vi "compress_parameters_1.vi"(2 "analog parameters":dbl[](array[numeric]), 3 "AI table":string[](array[string]), 4 "date/time string":string, 5 "table":string) -> (0 "Data to write":bool, 1 "parameters":string)   [LabVIEW 2019, in "PostgreSQL.lvlib"]
uses:
  PostgreSQL.lvlib
panel:
  in  "default string":string="INSERT INTO public.\"XX00.XX00.XX00.XX00.XX00_XQ.7001\"\n (\"time\", \"XX00XX00XX00XX00XX000000_XQ01\", \"XX00XX00XX00XX00XX000001_XQ01\", \"XX00XX00XX00XX00XX000002_XQ01\", \"XX00XX00XX00XX00XX000003_XQ01\", \"XX00XX00XX00XX00XX000004_XQ01\", \"XX00XX00XX00XX00XX000005_XQ01\", \"XX00XX00XX00XX00XX000006_XQ01\", \"XX00XX00XX00XX00XX000007_XQ01\", \"XX00XX00XX00XX00XX000008_XQ01\", \"XX00XX00XX00XX00XX000009_XQ01\", \"XX00XX00XX00XX00XX000010_XQ01\", \"XX00XX00XX00XX00XX000011_XQ01\", \"XX00XX00XX00XX00XX000012_XQ01\", \"XX00XX00XX00XX00XX000013_XQ01\", \"XX00XX00XX00XX00XX000014_XQ01\", \"XX00XX00XX00XX00XX000015_XQ01\", \"XX00XX00XX00XX00XX000016_XQ01\", \"XX00XX00XX00XX00XX000017_XQ01\", \"XX00XX00XX00XX00XX000018_XQ01\", \"XX00XX00XX00XX00XX000019_XQ01\", \"XX00XX00XX00XX00XX000020_XQ01\", \"XX00XX00XX00XX00XX000021_XQ01\", \"XX00XX00XX00XX00XX000022_XQ01\", \"XX00XX00XX00XX00XX000023_XQ01\", \"XX00XX00XX00XX00XX000024_XQ01\", \"XX00XX00XX00XX00XX000025_XQ01\", \"XX00XX00XX00XX00XX000026_XQ01\", \"XX00XX00XX00XX00XX000027_XQ01\", \"XX00XX00XX00XX00XX000028_XQ01\", \"XX00XX00XX00XX00XX000029_XQ01\", \"XX00XX00XX00XX00XX000030_XQ01\", \"XX00XX00XX00XX00XX000031_XQ01\", \"XX00XX00XX00XX00XX000032_XQ01\", \"XX00XX00XX00XX00XX000033_XQ01\", \"XX00XX00XX00XX00XX000034_XQ01\", \"XX00XX00XX00XX00XX000035_XQ01\", \"XX00XX00XX00XX00XX000036_XQ01\", \"XX00XX00XX00XX00XX000037_XQ01\", \"XX00XX00XX00XX00XX000038_XQ01\", \"XX00XX00XX00XX00XX000039_XQ01\", \"XX00XX00XX00XX00XX000040_XQ01\", \"XX00XX00XX00XX00XX000041_XQ01\", \"XX00XX00XX00XX00XX000042_XQ01\", \"XX00XX00XX00XX00XX000043_XQ01\", \"XX00XX00XX00XX00XX000044_XQ01\", \"XX00XX00XX00XX00XX000045_XQ01\", \"XX00XX00XX00XX00XX000046_XQ01\", \"XX00XX00XX00XX00XX000047_XQ01\", \"XX00XX00XX00XX00XX000048_XQ01\", \"XX00XX00XX00XX00XX000049_XQ01\", \"XX00XX00XX00XX00XX000050_XQ01\", \"XX00XX00XX00XX00XX000051_XQ01\", \"XX00XX00XX00XX00XX000052_XQ01\", \"XX00XX00XX00XX00XX000053_XQ01\", \"XX00XX00XX00XX00XX000054_XQ01\", \"XX00XX00XX00XX00XX000055_XQ01\", \"XX00XX00XX00XX00XX000056_XQ01\", \"XX00XX00XX00XX00XX000057_XQ01\", \"XX00XX00XX00XX00XX000058_XQ01\", \"XX00XX00XX00XX00XX000059_XQ01\", \"XX00XX00XX00XX00XX000060_XQ01\", \"XX00XX00XX00XX00XX000061_XQ01\", \"XX00XX00XX00XX00XX000062_XQ01\", \"XX00XX00XX00XX00XX000063_XQ01\", \"XX00XX00XX00XX00XX000064_XQ01\", \"XX00XX00XX00XX00XX000065_XQ01\", \"XX00XX00XX00XX00XX000066_XQ01\", \"XX00XX00XX00XX00XX000067_XQ01\", \"XX00XX00XX00XX00XX000068_XQ01\", \"XX00XX00XX00XX00XX000069_XQ01\", \"XX00XX00XX00XX00XX000070_XQ01\", \"XX00XX00XX00XX00XX000071_XQ01\", \"XX00XX00XX00XX00XX000072_XQ01\", \"XX00XX00XX00XX00XX000073_XQ01\", \"XX00XX00XX00XX00XX000074_XQ01\", \"XX00XX00XX00XX00XX000075_XQ01\", \"XX00XX00XX00XX00XX000076_XQ01\", \"XX00XX00XX00XX00XX000077_XQ01\", \"XX00XX00XX00XX00XX000078_XQ01\", \"XX00XX00XX00XX00XX000079_XQ01\", \"XX00XX00XX00XX00XX000080_XQ01\", \"XX00XX00XX00XX00XX000081_XQ01\", \"XX00XX00XX00XX00XX000082_XQ01\", \"XX00XX00XX00XX00XX000083_XQ01\", \"XX00XX00XX00XX00XX000084_XQ01\", \"XX00XX00XX00XX00XX000085_XQ01\", \"XX00XX00XX00XX00XX000086_XQ01\", \"XX00XX00XX00XX00XX000087_XQ01\", \"XX00XX00XX00XX00XX000088_XQ01\", \"XX00XX00XX00XX00XX000089_XQ01\", \"XX00XX00XX00XX00XX000090_XQ01\", \"XX00XX00XX00XX00XX000091_XQ01\", \"XX00XX00XX00XX00XX000092_XQ01\", \"XX00XX00XX00XX00XX000093_XQ01\", \"XX00XX00XX00XX00XX000094_XQ01\", \"XX00XX00XX00XX00XX000095_XQ01\", \"XX00XX00XX00XX00XX000096_XQ01\", \"XX00XX00XX00XX00XX000097_XQ01\", \"XX00XX00XX00XX00XX000098_XQ01\", \"XX00XX00XX00XX00XX000099_XQ01\", \"XX00XX00XX00XX00XX000100_XQ01\", \"XX00XX00XX00XX00XX000101_XQ01\", \"XX00XX00XX00XX00XX000102_XQ01\", \"XX00XX00XX00XX00XX000103_XQ01\", \"XX00XX00XX00XX00XX000104_XQ01\", \"XX00XX00XX00XX00XX000105_XQ01\", \"XX00XX00XX00XX00XX000106_XQ01\", \"XX00XX00XX00XX00XX000107_XQ01\", \"XX00XX00XX00XX00XX000108_XQ01\", \"XX00XX00XX00XX00XX000109_XQ01\", \"XX00XX00XX00XX00XX000110_XQ01\", \"XX00XX00XX00XX00XX000111_XQ01\", \"XX00XX00XX00XX00XX000112_XQ01\", \"XX00XX00XX00XX00XX000113_XQ01\", \"XX00XX00XX00XX00XX000114_XQ01\", \"XX00XX00XX00XX00XX000115_XQ01\", \"XX00XX00XX00XX00XX000116_XQ01\", \"XX00XX00XX00XX00XX000117_XQ01\", \"XX00XX00XX00XX00XX000118_XQ01\", \"XX00XX00XX00XX00XX000119_XQ01\", \"XX00XX00XX00XX00XX000120_XQ01\", \"XX00XX00XX00XX00XX000121_XQ01\", \"XX00XX00XX00XX00XX000122_XQ01\", \"XX00XX00XX00XX00XX000123_XQ01\", \"XX00XX00XX00XX00XX000124_XQ01\", \"XX00XX00XX00XX00XX000125_XQ01\", \"XX00XX00XX00XX00XX000126_XQ01\", \"XX00XX00XX00XX00XX000127_XQ01\", \"XX00XX00XX00XX00XX000128_XQ01\", \"XX00XX00XX00XX00XX000129_XQ01\", \"XX00XX00XX00XX00XX000130_XQ01\", \"XX00XX00XX00XX00XX000131_XQ01\", \"XX00XX00XX00XX00XX000132_XQ01\", \"XX00XX00XX00XX00XX000133_XQ01\", \"XX00XX00XX00XX00XX000134_XQ01\", \"XX00XX00XX00XX00XX000135_XQ01\", \"XX00XX00XX00XX00XX000136_XQ01\", \"XX00XX00XX00XX00XX000137_XQ01\", \"XX00XX00XX00XX00XX000138_XQ01\", \"XX00XX00XX00XX00XX000139_XQ01\", \"XX00XX00XX00XX00XX000140_XQ01\", \"XX00XX00XX00XX00XX000141_XQ01\", \"XX00XX00XX00XX00XX000142_XQ01\", \"XX00XX00XX00XX00XX000143_XQ01\", \"XX00XX00XX00XX00XX000144_XQ01\", \"XX00XX00XX00XX00XX000145_XQ01\", \"XX00XX00XX00XX00XX000146_XQ01\", \"XX00XX00XX00XX00XX000147_XQ01\", \"XX00XX00XX00XX00XX000148_XQ01\", \"XX00XX00XX00XX00XX000149_XQ01\", \"XX00XX00XX00XX00XX000150_XQ01\", \"XX00XX00XX00XX00XX000151_XQ01\", \"XX00XX00XX00XX00XX000152_XQ01\", \"XX00XX00XX00XX00XX000153_XQ01\", \"XX00XX00XX00XX00XX000154_XQ01\", \"XX00XX00XX00XX00XX000155_XQ01\", \"XX00XX00XX00XX00XX000156_XQ01\", \"XX00XX00XX00XX00XX000157_XQ01\", \"XX00XX00XX00XX00XX000158_XQ01\", \"XX00XX00XX00XX00XX000159_XQ01\", \"XX00XX00XX00XX00XX000160_XQ01\", \"XX00XX00XX00XX00XX000161_XQ01\", \"XX00XX00XX00XX00XX000162_XQ01\", \"XX00XX00XX00XX00XX000163_XQ01\", \"XX00XX00XX00XX00XX000164_XQ01\", \"XX00XX00XX00XX00XX000165_XQ01\", \"XX00XX00XX00XX00XX000166_XQ01\", \"XX00XX00XX00XX00XX000167_XQ01\", \"XX00XX00XX00XX00XX000168_XQ01\", \"XX00XX00XX00XX00XX000169_XQ01\", \"XX00XX00XX00XX00XX000170_XQ01\", \"XX00XX00XX00XX00XX000171_XQ01\", \"XX00XX00XX00XX00XX000172_XQ01\", \"XX00XX00XX00XX00XX000173_XQ01\", \"XX00XX00XX00XX00XX000174_XQ01\", \"XX00XX00XX00XX00XX000175_XQ01\", \"XX00XX00XX00XX00XX000176_XQ01\", \"XX00XX00XX00XX00XX000177_XQ01\", \"XX00XX00XX00XX00XX000178_XQ01\", \"XX00XX00XX00XX00XX000179_XQ01\", \"XX00XX00XX00XX00XX000180_XQ01\", \"XX00XX00XX00XX00XX000181_XQ01\", \"XX00XX00XX00XX00XX000182_XQ01\", \"XX00XX00XX00XX00XX000183_XQ01\", \"XX00XX00XX00XX00XX000184_XQ01\", \"XX00XX00XX00XX00XX000185_XQ01\", \"XX00XX00XX00XX00XX000186_XQ01\", \"XX00XX00XX00XX00XX000187_XQ01\", \"XX00XX00XX00XX00XX000188_XQ01\", \"XX00XX00XX00XX00XX000189_XQ01\", \"XX00XX00XX00XX00XX000190_XQ01\", \"XX00XX00XX00XX00XX000191_XQ01\", \"XX00XX00XX00XX00XX000192_XQ01\", \"XX00XX00XX00XX00XX000193_XQ01\", \"XX00XX00XX00XX00XX000194_XQ01\", \"XX00XX00XX00XX00XX000195_XQ01\", \"XX00XX00XX00XX00XX000196_XQ01\", \"XX00XX00XX00XX00XX000197_XQ01\", \"XX00XX00XX00XX00XX000198_XQ01\", \"XX00XX00XX00XX00XX000199_XQ01\", \"XX00XX00XX00XX00XX000200_XQ01\", \"XX00XX00XX00XX00XX000201_XQ01\", \"XX00XX00XX00XX00XX000202_XQ01\", \"XX00XX00XX00XX00XX000203_XQ01\", \"XX00XX00XX00XX00XX000204_XQ01\", \"XX00XX00XX00XX00XX000205_XQ01\", \"XX00XX00XX00XX00XX000206_XQ01\", \"XX00XX00XX00XX00XX000207_XQ01\", \"XX00XX00XX00XX00XX000208_XQ01\", \"XX00XX00XX00XX00XX000209_XQ01\", \"XX00XX00XX00XX00XX000210_XQ01\", \"XX00XX00XX00XX00XX000211_XQ01\", \"XX00XX00XX00XX00XX000212_XQ01\", \"XX00XX00XX00XX00XX000213_XQ01\", \"XX00XX00XX00XX00XX000214_XQ01\", \"XX00XX00XX00XX00XX000215_XQ01\", \"XX00XX00XX00XX00XX000216_XQ01\", \"XX00XX00XX00XX00XX000217_XQ01\", \"XX00XX00XX00XX00XX000218_XQ01\", \"XX00XX00XX00XX00XX000219_XQ01\", \"XX00XX00XX00XX00XX000220_XQ01\", \"XX00XX00XX00XX00XX000221_XQ01\", \"XX00XX00XX00XX00XX000222_XQ01\", \"XX00XX00XX00XX00XX000223_XQ01\", \"XX00XX00XX00XX00XX000224_XQ01\", \"XX00XX00XX00XX00XX000225_XQ01\", \"XX00XX00XX00XX00XX000226_XQ01\", \"XX00XX00XX00XX00XX000227_XQ01\", \"XX00XX00XX00XX00XX000228_XQ01\", \"XX00XX00XX00XX00XX000229_XQ01\", \"XX00XX00XX00XX00XX000230_XQ01\", \"XX00XX00XX00XX00XX000231_XQ01\", \"XX00XX00XX00XX00XX000232_XQ01\", \"XX00XX00XX00XX00XX000233_XQ01\", \"XX00XX00XX00XX00XX000234_XQ01\", \"XX00XX00XX00XX00XX000235_XQ01\", \"XX00XX00XX00XX00XX000236_XQ01\", \"XX00XX00XX00XX00XX000237_XQ01\", \"XX00XX00XX00XX00XX000238_XQ01\", \"XX00XX00XX00XX00XX000239_XQ01\", \"XX00XX00XX00XX00XX000240_XQ01\", \"XX00XX00XX00XX00XX000241_XQ01\", \"XX00XX00XX00XX00XX000242_XQ01\", \"XX00XX00XX00XX00XX000243_XQ01\", \"XX00XX00XX00XX00XX000244_XQ01\", \"XX00XX00XX00XX00XX000245_XQ01\", \"XX00XX00XX00XX00XX000246_XQ01\", \"XX00XX00XX00XX00XX000247_XQ01\", \"XX00XX00XX00XX00XX000248_XQ01\", \"XX00XX00XX00XX00XX000249_XQ01\", \"XX00XX00XX00XX00XX000250_XQ01\", \"XX00XX00XX00XX00XX000251_XQ01\", \"XX00XX00XX00XX00XX000252_XQ01\", \"XX00XX00XX00XX00XX000253_XQ01\", \"XX00XX00XX00XX00XX000254_XQ01\", \"XX00XX00XX00XX00XX000255_XQ01\", \"XX00XX00XX00XX00XX000256_XQ01\", \"XX00XX00XX00XX00XX000257_XQ01\", \"XX00XX00XX00XX00XX000258_XQ01\", \"XX00XX00XX00XX00XX000259_XQ01\", \"XX00XX00XX00XX00XX000260_XQ01\", \"XX00XX00XX00XX00XX000261_XQ01\", \"XX00XX00XX00XX00XX000262_XQ01\", \"XX00XX00XX00XX00XX000263_XQ01\", \"XX00XX00XX00XX00XX000264_XQ01\", \"XX00XX00XX00XX00XX000265_XQ01\", \"XX00XX00XX00XX00XX000266_XQ01\", \"XX00XX00XX00XX00XX000267_XQ01\", \"XX00XX00XX00XX00XX000268_XQ01\", \"XX00XX00XX00XX00XX000269_XQ01\", \"XX00XX00XX00XX00XX000270_XQ01\", \"XX00XX00XX00XX00XX000271_XQ01\", \"XX00XX00XX00XX00XX000272_XQ01\", \"XX00XX00XX00XX00XX000273_XQ01\", \"XX00XX00XX00XX00XX000274_XQ01\", \"XX00XX00XX00XX00XX000275_XQ01\", \"XX00XX00XX00XX00XX000276_XQ01\", \"XX00XX00XX00XX00XX000277_XQ01\", \"XX00XX00XX00XX00XX000278_XQ01\", \"XX00XX00XX00XX00XX000279_XQ01\", \"XX00XX00XX00XX00XX000280_XQ01\", \"XX00XX00XX00XX00XX000281_XQ01\", \"XX00XX00XX00XX00XX000282_XQ01\", \"XX00XX00XX00XX00XX000283_XQ01\", \"XX00XX00XX00XX00XX000284_XQ01\", \"XX00XX00XX00XX00XX000285_XQ01\", \"XX00XX00XX00XX00XX000286_XQ01\", \"XX00XX00XX00XX00XX000287_XQ01\", \"XX00XX00XX00XX00XX000288_XQ01\", \"XX00XX00XX00XX00XX000289_XQ01\", \"XX00XX00XX00XX00XX000290_XQ01\", \"XX00XX00XX00XX00XX000291_XQ01\", \"XX00XX00XX00XX00XX000292_XQ01\", \"XX00XX00XX00XX00XX000293_XQ01\", \"XX00XX00XX00XX00XX000294_XQ01\", \"XX00XX00XX00XX00XX000295_XQ01\", \"XX00XX00XX00XX00XX000296_XQ01\", \"XX00XX00XX00XX00XX000297_XQ01\", \"XX00XX00XX00XX00XX000298_XQ01\", \"XX00XX00XX00XX00XX000299_XQ01\", \"XX00XX00XX00XX00XX000300_XQ01\", \"XX00XX00XX00XX00XX000301_XQ01\", \"XX00XX00XX00XX00XX000302_XQ01\", \"XX00XX00XX00XX00XX000303_XQ01\", \"XX00XX00XX00XX00XX000304_XQ01\", \"XX00XX00XX00XX00XX000305_XQ01\", \"XX00XX00XX00XX00XX000306_XQ01\", \"XX00XX00XX00XX00XX000307_XQ01\", \"XX00XX00XX00XX00XX000308_XQ01\", \"XX00XX00XX00XX00XX000309_XQ01\", \"XX00XX00XX00XX00XX000310_XQ01\", \"XX00XX00XX00XX00XX000311_XQ01\", \"XX00XX00XX00XX00XX000312_XQ01\", \"XX00XX00XX00XX00XX000313_XQ01\", \"XX00XX00XX00XX00XX000314_XQ01\", \"XX00XX00XX00XX00XX000315_XQ01\", \"XX00XX00XX00XX00XX000316_XQ01\", \"XX00XX00XX00XX00XX000317_XQ01\", \"XX00XX00XX00XX00XX000318_XQ01\", \"XX00XX00XX00XX00XX000319_XQ01\", \"XX00XX00XX00XX00XX000320_XQ01\", \"XX00XX00XX00XX00XX000321_XQ01\", \"XX00XX00XX00XX00XX000322_XQ01\", \"XX00XX00XX00XX00XX000323_XQ01\", \"XX00XX00XX00XX00XX000324_XQ01\", \"XX00XX00XX00XX00XX000325_XQ01\", \"XX00XX00XX00XX00XX000326_XQ01\", \"XX00XX00XX00XX00XX000327_XQ01\", \"XX00XX00XX00XX00XX000328_XQ01\", \"XX00XX00XX00XX00XX000329_XQ01\", \"XX00XX00XX00XX00XX000330_XQ01\", \"XX00XX00XX00XX00XX000331_XQ01\", \"XX00XX00XX00XX00XX000332_XQ01\", \"XX00XX00XX00XX00XX000333_XQ01\", \"XX00XX00XX00XX00XX000334_XQ01\", \"XX00XX00XX00XX00XX000335_XQ01\", \"XX00XX00XX00XX00XX000336_XQ01\", \"XX00XX00XX00XX00XX000337_XQ01\", \"XX00XX00XX00XX00XX000338_XQ01\", \"XX00XX00XX00XX00XX000339_XQ01\", \"XX00XX00XX00XX00XX000340_XQ01\", \"XX00XX00XX00XX00XX000341_XQ01\", \"XX00XX00XX00XX00XX000342_XQ01\", \"XX00XX00XX00XX00XX000343_XQ01\", \"XX00XX00XX00XX00XX000344_XQ01\", \"XX00XX00XX00XX00XX000345_XQ01\", \"XX00XX00XX00XX00XX000346_XQ01\", \"XX00XX00XX00XX00XX000347_XQ01\", \"XX00XX00XX00XX00XX000348_XQ01\", \"XX00XX00XX00XX00XX000349_XQ01\", \"XX00XX00XX00XX00XX000350_XQ01\", \"XX00XX00XX00XX00XX000351_XQ01\", \"XX00XX00XX00XX00XX000352_XQ01\", \"XX00XX00XX00XX00XX000353_XQ01\", \"XX00XX00XX00XX00XX000354_XQ01\", \"XX00XX00XX00XX00XX000355_XQ01\", \"XX00XX00XX00XX00XX000356_XQ01\", \"XX00XX00XX00XX00XX000357_XQ01\", \"XX00XX00XX00XX00XX000358_XQ01\", \"XX00XX00XX00XX00XX000359_XQ01\", \"XX00XX00XX00XX00XX000360_XQ01\", \"XX00XX00XX00XX00XX000361_XQ01\", \"XX00XX00XX00XX00XX000362_XQ01\", \"XX00XX00XX00XX00XX000363_XQ01\", \"XX00XX00XX00XX00XX000364_XQ01\", \"XX00XX00XX00XX00XX000365_XQ01\", \"XX00XX00XX00XX00XX000366_XQ01\", \"XX00XX00XX00XX00XX000367_XQ01\", \"XX00XX00XX00XX00XX000368_XQ01\", \"XX00XX00XX00XX00XX000369_XQ01\", \"XX00XX00XX00XX00XX000370_XQ01\", \"XX00XX00XX00XX00XX000371_XQ01\", \"XX00XX00XX00XX00XX000372_XQ01\", \"XX00XX00XX00XX00XX000373_XQ01\", \"XX00XX00XX00XX00XX000374_XQ01\", \"XX00XX00XX00XX00XX000375_XQ01\", \"XX00XX00XX00XX00XX000376_XQ01\", \"XX00XX00XX00XX00XX000377_XQ01\", \"XX00XX00XX00XX00XX000378_XQ01\", \"XX00XX00XX00XX00XX000379_XQ01\", \"XX00XX00XX00XX00XX000380_XQ01\", \"XX00XX00XX00XX00XX000381_XQ01\", \"XX00XX00XX00XX00XX000382_XQ01\", \"XX00XX00XX00XX00XX000383_XQ01\", \"XX00XX00XX00XX00XX000384_XQ01\", \"XX00XX00XX00XX00XX000385_XQ01\", \"XX00XX00XX00XX00XX000386_XQ01\", \"XX00XX00XX00XX00XX000387_XQ01\", \"XX00XX00XX00XX00XX000388_XQ01\", \"XX00XX00XX00XX00XX000389_XQ01\", \"XX00XX00XX00XX00XX000390_XQ01\", \"XX00XX00XX00XX00XX000391_XQ01\", \"XX00XX00XX00XX00XX000392_XQ01\", \"XX00XX00XX00XX00XX000393_XQ01\", \"XX00XX00XX00XX00XX000394_XQ01\", \"XX00XX00XX00XX00XX000395_XQ01\", \"XX00XX00XX00XX00XX000396_XQ01\", \"XX00XX00XX00XX00XX000397_XQ01\", \"XX00XX00XX00XX00XX000398_XQ01\", \"XX00XX00XX00XX00XX000399_XQ01\", \"XX00XX00XX00XX00XX000400_XQ01\", \"XX00XX00XX00XX00XX000401_XQ01\", \"XX00XX00XX00XX00XX000402_XQ01\", \"XX00XX00XX00XX00XX000403_XQ01\", \"XX00XX00XX00XX00XX000404_XQ01\", \"XX00XX00XX00XX00XX000405_XQ01\", \"XX00XX00XX00XX00XX000406_XQ01\", \"XX00XX00XX00XX00XX000407_XQ01\", \"XX00XX00XX00XX00XX000408_XQ01\", \"XX00XX00XX00XX00XX000409_XQ01\", \"XX00XX00XX00XX00XX000410_XQ01\", \"XX00XX00XX00XX00XX000411_XQ01\", \"XX00XX00XX00XX00XX000412_XQ01\", \"XX00XX00XX00XX00XX000413_XQ01\", \"XX00XX00XX00XX00XX000414_XQ01\", \"XX00XX00XX00XX00XX000415_XQ01\", \"XX00XX00XX00XX00XX000416_XQ01\", \"XX00XX00XX00XX00XX000417_XQ01\", \"XX00XX00XX00XX00XX000418_XQ01\", \"XX00XX00XX00XX00XX000419_XQ01\", \"XX00XX00XX00XX00XX000420_XQ01\", \"XX00XX00XX00XX00XX000421_XQ01\", \"XX00XX00XX00XX00XX000422_XQ01\", \"XX00XX00XX00XX00XX000423_XQ01\", \"XX00XX00XX00XX00XX000424_XQ01\", \"XX00XX00XX00XX00XX000425_XQ01\", \"XX00XX00XX00XX00XX000426_XQ01\", \"XX00XX00XX00XX00XX000427_XQ01\", \"XX00XX00XX00XX00XX000428_XQ01\", \"XX00XX00XX00XX00XX000429_XQ01\", \"XX00XX00XX00XX00XX000430_XQ01\", \"XX00XX00XX00XX00XX000431_XQ01\", \"XX00XX00XX00XX00XX000432_XQ01\", \"XX00XX00XX00XX00XX000433_XQ01\", \"XX00XX00XX00XX00XX000434_XQ01\", \"XX00XX00XX00XX00XX000435_XQ01\", \"XX00XX00XX00XX00XX000436_XQ01\", \"XX00XX00XX00XX00XX000437_XQ01\", \"XX00XX00XX00XX00XX000438_XQ01\", \"XX00XX00XX00XX00XX000439_XQ01\", \"XX00XX00XX00XX00XX000440_XQ01\", \"XX00XX00XX00XX00XX000441_XQ01\", \"XX00XX00XX00XX00XX000442_XQ01\", \"XX00XX00XX00XX00XX000443_XQ01\", \"XX00XX00XX00XX00XX000444_XQ01\", \"XX00XX00XX00XX00XX000445_XQ01\", \"XX00XX00XX00XX00XX000446_XQ01\", \"XX00XX00XX00XX00XX000447_XQ01\", \"XX00XX00XX00XX00XX000448_XQ01\", \"XX00XX00XX00XX00XX000449_XQ01\", \"XX00XX00XX00XX00XX000450_XQ01\", \"XX00XX00XX00XX00XX000451_XQ01\", \"XX00XX00XX00XX00XX000452_XQ01\", \"XX00XX00XX00XX00XX000453_XQ01\", \"XX00XX00XX00XX00XX000454_XQ01\", \"XX00XX00XX00XX00XX000455_XQ01\", \"XX00XX00XX00XX00XX000456_XQ01\", \"XX00XX00XX00XX00XX000457_XQ01\", \"XX00XX00XX00XX00XX000458_XQ01\", \"XX00XX00XX00XX00XX000459_XQ01\", \"XX00XX00XX00XX00XX000460_XQ01\", \"XX00XX00XX00XX00XX000461_XQ01\", \"XX00XX00XX00XX00XX000462_XQ01\", \"XX00XX00XX00XX00XX000463_XQ01\", \"XX00XX00XX00XX00XX000464_XQ01\", \"XX00XX00XX00XX00XX000465_XQ01\", \"XX00XX00XX00XX00XX000466_XQ01\", \"XX00XX00XX00XX00XX000467_XQ01\", \"XX00XX00XX00XX00XX000468_XQ01\", \"XX00XX00XX00XX00XX000469_XQ01\", \"XX00XX00XX00XX00XX000470_XQ01\", \"XX00XX00XX00XX00XX000471_XQ01\", \"XX00XX00XX00XX00XX000472_XQ01\", \"XX00XX00XX00XX00XX000473_XQ01\", \"XX00XX00XX00XX00XX000474_XQ01\", \"XX00XX00XX00XX00XX000475_XQ01\", \"XX00XX00XX00XX00XX000476_XQ01\", \"XX00XX00XX00XX00XX000477_XQ01\", \"XX00XX00XX00XX00XX000478_XQ01\", \"XX00XX00XX00XX00XX000479_XQ01\", \"XX00XX00XX00XX00XX000480_XQ01\", \"XX00XX00XX00XX00XX000481_XQ01\", \"XX00XX00XX00XX00XX000482_XQ01\", \"XX00XX00XX00XX00XX000483_XQ01\", \"XX00XX00XX00XX00XX000484_XQ01\", \"XX00XX00XX00XX00XX000485_XQ01\", \"XX00XX00XX00XX00XX000486_XQ01\", \"XX00XX00XX00XX00XX000487_XQ01\", \"XX00XX00XX00XX00XX000488_XQ01\", \"XX00XX00XX00XX00XX000489_XQ01\", \"XX00XX00XX00XX00XX000490_XQ01\", \"XX00XX00XX00XX00XX000491_XQ01\", \"XX00XX00XX00XX00XX000492_XQ01\", \"XX00XX00XX00XX00XX000493_XQ01\", \"XX00XX00XX00XX00XX000494_XQ01\", \"XX00XX00XX00XX00XX000495_XQ01\", \"XX00XX00XX00XX00XX000496_XQ01\", \"XX00XX00XX00XX00XX000497_XQ01\", \"XX00XX00XX00XX00XX000498_XQ01\", \"XX00XX00XX00XX00XX000499_XQ01\", \"XX00XX00XX00XX00XX000500_XQ01\", \"XX00XX00XX00XX00XX000501_XQ01\", \"XX00XX00XX00XX00XX000502_XQ01\", \"XX00XX00XX00XX00XX000503_XQ01\", \"XX00XX00XX00XX00XX000504_XQ01\", \"XX00XX00XX00XX00XX000505_XQ01\", \"XX00XX00XX00XX00XX000506_XQ01\", \"XX00XX00XX00XX00XX000507_XQ01\", \"XX00XX00XX00XX00XX000508_XQ01\", \"XX00XX00XX00XX00XX000509_XQ01\", \"XX00XX00XX00XX00XX000510_XQ01\", \"XX00XX00XX00XX00XX000511_XQ01\", \"XX00XX00XX00XX00XX000512_XQ01\", \"XX00XX00XX00XX00XX000513_XQ01\", \"XX00XX00XX00XX00XX000514_XQ01\", \"XX00XX00XX00XX00XX000515_XQ01\", \"XX00XX00XX00XX00XX000516_XQ01\", \"XX00XX00XX00XX00XX000517_XQ01\", \"XX00XX00XX00XX00XX000518_XQ01\", \"XX00XX00XX00XX00XX000519_XQ01\", \"XX00XX00XX00XX00XX000520_XQ01\", \"XX00XX00XX00XX00XX000521_XQ01\", \"XX00XX00XX00XX00XX000522_XQ01\", \"XX00XX00XX00XX00XX000523_XQ01\", \"XX00XX00XX00XX00XX000524_XQ01\", \"XX00XX00XX00XX00XX000525_XQ01\", \"XX00XX00XX00XX00XX000526_XQ01\", \"XX00XX00XX00XX00XX000527_XQ01\", \"XX00XX00XX00XX00XX000528_XQ01\", \"XX00XX00XX00XX00XX000529_XQ01\", \"XX00XX00XX00XX00XX000530_XQ01\", \"XX00XX00XX00XX00XX000531_XQ01\", \"XX00XX00XX00XX00XX000532_XQ01\", \"XX00XX00XX00XX00XX000533_XQ01\", \"XX00XX00XX00XX00XX000534_XQ01\", \"XX00XX00XX00XX00XX000535_XQ01\", \"XX00XX00XX00XX00XX000536_XQ01\", \"XX00XX00XX00XX00XX000537_XQ01\", \"XX00XX00XX00XX00XX000538_XQ01\", \"XX00XX00XX00XX00XX000539_XQ01\", \"XX00XX00XX00XX00XX000540_XQ01\", \"XX00XX00XX00XX00XX000541_XQ01\", \"XX00XX00XX00XX00XX000542_XQ01\", \"XX00XX00XX00XX00XX000543_XQ01\", \"XX00XX00XX00XX00XX000544_XQ01\", \"XX00XX00XX00XX00XX000545_XQ01\", \"XX00XX00XX00XX00XX000546_XQ01\", \"XX00XX00XX00XX00XX000547_XQ01\", \"XX00XX00XX00XX00XX000548_XQ01\", \"XX00XX00XX00XX00XX000549_XQ01\", \"XX00XX00XX00XX00XX000550_XQ01\", \"XX00XX00XX00XX00XX000551_XQ01\", \"XX00XX00XX00XX00XX000552_XQ01\", \"XX00XX00XX00XX00XX000553_XQ01\", \"XX00XX00XX00XX00XX000554_XQ01\", \"XX00XX00XX00XX00XX000555_XQ01\", \"XX00XX00XX00XX00XX000556_XQ01\", \"XX00XX00XX00XX00XX000557_XQ01\", \"XX00XX00XX00XX00XX000558_XQ01\", \"XX00XX00XX00XX00XX000559_XQ01\", \"XX00XX00XX00XX00XX000560_XQ01\", \"XX00XX00XX00XX00XX000561_XQ01\", \"XX00XX00XX00XX00XX000562_XQ01\", \"XX00XX00XX00XX00XX000563_XQ01\", \"XX00XX00XX00XX00XX000564_XQ01\", \"XX00XX00XX00XX00XX000565_XQ01\", \"XX00XX00XX00XX00XX000566_XQ01\", \"XX00XX00XX00XX00XX000567_XQ01\", \"XX00XX00XX00XX00XX000568_XQ01\", \"XX00XX00XX00XX00XX000569_XQ01\", \"XX00XX00XX00XX00XX000570_XQ01\", \"XX00XX00XX00XX00XX000571_XQ01\", \"XX00XX00XX00XX00XX000572_XQ01\", \"XX00XX00XX00XX00XX000573_XQ01\", \"XX00XX00XX00XX00XX000574_XQ01\", \"XX00XX00XX00XX00XX000575_XQ01\", \"XX00XX00XX00XX00XX000576_XQ01\", \"XX00XX00XX00XX00XX000577_XQ01\", \"XX00XX00XX00XX00XX000578_XQ01\", \"XX00XX00XX00XX00XX000579_XQ01\", \"XX00XX00XX00XX00XX000580_XQ01\", \"XX00XX00XX00XX00XX000581_XQ01\", \"XX00XX00XX00XX00XX000582_XQ01\", \"XX00XX00XX00XX00XX000583_XQ01\", \"XX00XX00XX00XX00XX000584_XQ01\", \"XX00XX00XX00XX00XX000585_XQ01\", \"XX00XX00XX00XX00XX000586_XQ01\", \"XX00XX00XX00XX00XX000587_XQ01\", \"XX00XX00XX00XX00XX000588_XQ01\", \"XX00XX00XX00XX00XX000589_XQ01\", \"XX00XX00XX00XX00XX000590_XQ01\", \"XX00XX00XX00XX00XX000591_XQ01\", \"XX00XX00XX00XX00XX000592_XQ01\", \"XX00XX00XX00XX00XX000593_XQ01\", \"XX00XX00XX00XX00XX000594_XQ01\", \"XX00XX00XX00XX00XX000595_XQ01\", \"XX00XX00XX00XX00XX000596_XQ01\", \"XX00XX00XX00XX00XX000597_XQ01\", \"XX00XX00XX00XX00XX000598_XQ01\", \"XX00XX00XX00XX00XX000599_XQ01\", \"XX00XX00XX00XX00XX000600_XQ01\", \"XX00XX00XX00XX00XX000601_XQ01\", \"XX00XX00XX00XX00XX000602_XQ01\", \"XX00XX00XX00XX00XX000603_XQ01\", \"XX00XX00XX00XX00XX000604_XQ01\", \"XX00XX00XX00XX00XX000605_XQ01\", \"XX00XX00XX00XX00XX000606_XQ01\", \"XX00XX00XX00XX00XX000607_XQ01\", \"XX00XX00XX00XX00XX000608_XQ01\", \"XX00XX00XX00XX00XX000609_XQ01\", \"XX00XX00XX00XX00XX000610_XQ01\", \"XX00XX00XX00XX00XX000611_XQ01\", \"XX00XX00XX00XX00XX000612_XQ01\", \"XX00XX00XX00XX00XX000613_XQ01\", \"XX00XX00XX00XX00XX000614_XQ01\", \"XX00XX00XX00XX00XX000615_XQ01\", \"XX00XX00XX00XX00XX000616_XQ01\", \"XX00XX00XX00XX00XX000617_XQ01\", \"XX00XX00XX00XX00XX000618_XQ01\", \"XX00XX00XX00XX00XX000619_XQ01\", \"XX00XX00XX00XX00XX000620_XQ01\", \"XX00XX00XX00XX00XX000621_XQ01\", \"XX00XX00XX00XX00XX000622_XQ01\", \"XX00XX00XX00XX00XX000623_XQ01\", \"XX00XX00XX00XX00XX000624_XQ01\", \"XX00XX00XX00XX00XX000625_XQ01\", \"XX00XX00XX00XX00XX000626_XQ01\", \"XX00XX00XX00XX00XX000627_XQ01\", \"XX00XX00XX00XX00XX000628_XQ01\", \"XX00XX00XX00XX00XX000629_XQ01\", \"XX00XX00XX00XX00XX000630_XQ01\", \"XX00XX00XX00XX00XX000631_XQ01\", \"XX00XX00XX00XX00XX000632_XQ01\", \"XX00XX00XX00XX00XX000633_XQ01\", \"XX00XX00XX00XX00XX000634_XQ01\", \"XX00XX00XX00XX00XX000635_XQ01\", \"XX00XX00XX00XX00XX000636_XQ01\", \"XX00XX00XX00XX00XX000637_XQ01\", \"XX00XX00XX00XX00XX000638_XQ01\", \"XX00XX00XX00XX00XX000639_XQ01\", \"XX00XX00XX00XX00XX000640_XQ01\", \"XX00XX00XX00XX00XX000641_XQ01\", \"XX00XX00XX00XX00XX000642_XQ01\", \"XX00XX00XX00XX00XX000643_XQ01\", \"XX00XX00XX00XX00XX000644_XQ01\", \"XX00XX00XX00XX00XX000645_XQ01\", \"XX00XX00XX00XX00XX000646_XQ01\", \"XX00XX00XX00XX00XX000647_XQ01\", \"XX00XX00XX00XX00XX000648_XQ01\", \"XX00XX00XX00XX00XX000649_XQ01\", \"XX00XX00XX00XX00XX000650_XQ01\", \"XX00XX00XX00XX00XX000651_XQ01\", \"XX00XX00XX00XX00XX000652_XQ01\", \"XX00XX00XX00XX00XX000653_XQ01\", \"XX00XX00XX00XX00XX000654_XQ01\", \"XX00XX00XX00XX00XX000655_XQ01\", \"XX00XX00XX00XX00XX000656_XQ01\", \"XX00XX00XX00XX00XX000657_XQ01\", \"XX00XX00XX00XX00XX000658_XQ01\", \"XX00XX00XX00XX00XX000659_XQ01\", \"XX00XX00XX00XX00XX000660_XQ01\", \"XX00XX00XX00XX00XX000661_XQ01\", \"XX00XX00XX00XX00XX000662_XQ01\", \"XX00XX00XX00XX00XX000663_XQ01\", \"XX00XX00XX00XX00XX000664_XQ01\", \"XX00XX00XX00XX00XX000665_XQ01\", \"XX00XX00XX00XX00XX000666_XQ01\", \"XX00XX00XX00XX00XX000667_XQ01\", \"XX00XX00XX00XX00XX000668_XQ01\", \"XX00XX00XX00XX00XX000669_XQ01\", \"XX00XX00XX00XX00XX000670_XQ01\", \"XX00XX00XX00XX00XX000671_XQ01\", \"XX00XX00XX00XX00XX000672_XQ01\", \"XX00XX00XX00XX00XX000673_XQ01\", \"XX00XX00XX00XX00XX000674_XQ01\", \"XX00XX00XX00XX00XX000675_XQ01\", \"XX00XX00XX00XX00XX000676_XQ01\", \"XX00XX00XX00XX00XX000677_XQ01\", \"XX00XX00XX00XX00XX000678_XQ01\", \"XX00XX00XX00XX00XX000679_XQ01\", \"XX00XX00XX00XX00XX000680_XQ01\", \"XX00XX00XX00XX00XX000681_XQ01\", \"XX00XX00XX00XX00XX000682_XQ01\", \"XX00XX00XX00XX00XX000683_XQ01\", \"XX00XX00XX00XX00XX000684_XQ01\", \"XX00XX00XX00XX00XX000685_XQ01\", \"XX00XX00XX00XX00XX000686_XQ01\", \"XX00XX00XX00XX00XX000687_XQ01\", \"XX00XX00XX00XX00XX000688_XQ01\", \"XX00XX00XX00XX00XX000689_XQ01\", \"XX00XX00XX00XX00XX000690_XQ01\", \"XX00XX00XX00XX00XX000691_XQ01\", \"XX00XX00XX00XX00XX000692_XQ01\", \"XX00XX00XX00XX00XX000693_XQ01\", \"XX00XX00XX00XX00XX000694_XQ01\", \"XX00XX00XX00XX00XX000695_XQ01\", \"XX00XX00XX00XX00XX000696_XQ01\", \"XX00XX00XX00XX00XX000697_XQ01\", \"XX00XX00XX00XX00XX000698_XQ01\", \"XX00XX00XX00XX00XX000699_XQ01\", \"XX00XX00XX00XX00XX000700_XQ01\", \"XX00XX00XX00XX00XX000701_XQ01\", \"XX00XX00XX00XX00XX000702_XQ01\", \"XX00XX00XX00XX00XX000703_XQ01\", \"XX00XX00XX00XX00XX000704_XQ01\", \"XX00XX00XX00XX00XX000705_XQ01\", \"XX00XX00XX00XX00XX000706_XQ01\", \"XX00XX00XX00XX00XX000707_XQ01\", \"XX00XX00XX00XX00XX000708_XQ01\", \"XX00XX00XX00XX00XX000709_XQ01\", \"XX00XX00XX00XX00XX000710_XQ01\", \"XX00XX00XX00XX00XX000711_XQ01\", \"XX00XX00XX00XX00XX000712_XQ01\", \"XX00XX00XX00XX00XX000713_XQ01\", \"XX00XX00XX00XX00XX000714_XQ01\", \"XX00XX00XX00XX00XX000715_XQ01\", \"XX00XX00XX00XX00XX000716_XQ01\", \"XX00XX00XX00XX00XX000717_XQ01\", \"XX00XX00XX00XX00XX000718_XQ01\", \"XX00XX00XX00XX00XX000719_XQ01\", \"XX00XX00XX00XX00XX000720_XQ01\", \"XX00XX00XX00XX00XX000721_XQ01\", \"XX00XX00XX00XX00XX000722_XQ01\", \"XX00XX00XX00XX00XX000723_XQ01\", \"XX00XX00XX00XX00XX000724_XQ01\", \"XX00XX00XX00XX00XX000725_XQ01\", \"XX00XX00XX00XX00XX000726_XQ01\", \"XX00XX00XX00XX00XX000727_XQ01\", \"XX00XX00XX00XX00XX000728_XQ01\", \"XX00XX00XX00XX00XX000729_XQ01\", \"XX00XX00XX00XX00XX000730_XQ01\", \"XX00XX00XX00XX00XX000731_XQ01\", \"XX00XX00XX00XX00XX000732_XQ01\", \"XX00XX00XX00XX00XX000733_XQ01\", \"XX00XX00XX00XX00XX000734_XQ01\", \"XX00XX00XX00XX00XX000735_XQ01\", \"XX00XX00XX00XX00XX000736_XQ01\", \"XX00XX00XX00XX00XX000737_XQ01\", \"XX00XX00XX00XX00XX000738_XQ01\", \"XX00XX00XX00XX00XX000739_XQ01\", \"XX00XX00XX00XX00XX000740_XQ01\", \"XX00XX00XX00XX00XX000741_XQ01\", \"XX00XX00XX00XX00XX000742_XQ01\", \"XX00XX00XX00XX00XX000743_XQ01\", \"XX00XX00XX00XX00XX000744_XQ01\", \"XX00XX00XX00XX00XX000745_XQ01\", \"XX00XX00XX00XX00XX000746_XQ01\", \"XX00XX00XX00XX00XX000747_XQ01\", \"XX00XX00XX00XX00XX000748_XQ01\", \"XX00XX00XX00XX00XX000749_XQ01\", \"XX00XX00XX00XX00XX000750_XQ01\", \"XX00XX00XX00XX00XX000751_XQ01\", \"XX00XX00XX00XX00XX000752_XQ01\", \"XX00XX00XX00XX00XX000753_XQ01\", \"XX00XX00XX00XX00XX000754_XQ01\", \"XX00XX00XX00XX00XX000755_XQ01\", \"XX00XX00XX00XX00XX000756_XQ01\", \"XX00XX00XX00XX00XX000757_XQ01\", \"XX00XX00XX00XX00XX000758_XQ01\", \"XX00XX00XX00XX00XX000759_XQ01\", \"XX00XX00XX00XX00XX000760_XQ01\", \"XX00XX00XX00XX00XX000761_XQ01\", \"XX00XX00XX00XX00XX000762_XQ01\", \"XX00XX00XX00XX00XX000763_XQ01\", \"XX00XX00XX00XX00XX000764_XQ01\", \"XX00XX00XX00XX00XX000765_XQ01\", \"XX00XX00XX00XX00XX000766_XQ01\", \"XX00XX00XX00XX00XX000767_XQ01\", \"XX00XX00XX00XX00XX000768_XQ01\", \"XX00XX00XX00XX00XX000769_XQ01\", \"XX00XX00XX00XX00XX000770_XQ01\", \"XX00XX00XX00XX00XX000771_XQ01\", \"XX00XX00XX00XX00XX000772_XQ01\", \"XX00XX00XX00XX00XX000773_XQ01\", \"XX00XX00XX00XX00XX000774_XQ01\", \"XX00XX00XX00XX00XX000775_XQ01\", \"XX00XX00XX00XX00XX000776_XQ01\", \"XX00XX00XX00XX00XX000777_XQ01\", \"XX00XX00XX00XX00XX000778_XQ01\", \"XX00XX00XX00XX00XX000779_XQ01\", \"XX00XX00XX00XX00XX000780_XQ01\", \"XX00XX00XX00XX00XX000781_XQ01\", \"XX00XX00XX00XX00XX000782_XQ01\", \"XX00XX00XX00XX00XX000783_XQ01\", \"XX00XX00XX00XX00XX000784_XQ01\", \"XX00XX00XX00XX00XX000785_XQ01\", \"XX00XX00XX00XX00XX000786_XQ01\", \"XX00XX00XX00XX00XX000787_XQ01\", \"XX00XX00XX00XX00XX000788_XQ01\", \"XX00XX00XX00XX00XX000789_XQ01\", \"XX00XX00XX00XX00XX000790_XQ01\", \"XX00XX00XX00XX00XX000791_XQ01\", \"XX00XX00XX00XX00XX000792_XQ01\", \"XX00XX00XX00XX00XX000793_XQ01\", \"XX00XX00XX00XX00XX000794_XQ01\", \"XX00XX00XX00XX00XX000795_XQ01\", \"XX00XX00XX00XX00XX000796_XQ01\", \"XX00XX00XX00XX00XX000797_XQ01\", \"XX00XX00XX00XX00XX000798_XQ01\", \"XX00XX00XX00XX00XX000799_XQ01\", \"XX00XX00XX00XX00XX000800_XQ01\", \"XX00XX00XX00XX00XX000801_XQ01\", \"XX00XX00XX00XX00XX000802_XQ01\", \"XX00XX00XX00XX00XX000803_XQ01\", \"XX00XX00XX00XX00XX000804_XQ01\", \"XX00XX00XX00XX00XX000805_XQ01\", \"XX00XX00XX00XX00XX000806_XQ01\", \"XX00XX00XX00XX00XX000807_XQ01\", \"XX00XX00XX00XX00XX000808_XQ01\", \"XX00XX00XX00XX00XX000809_XQ01\", \"XX00XX00XX00XX00XX000810_XQ01\", \"XX00XX00XX00XX00XX000811_XQ01\", \"XX00XX00XX00XX00XX000812_XQ01\", \"XX00XX00XX00XX00XX000813_XQ01\", \"XX00XX00XX00XX00XX000814_XQ01\", \"XX00XX00XX00XX00XX000815_XQ01\", \"XX00XX00XX00XX00XX000816_XQ01\", \"XX00XX00XX00XX00XX000817_XQ01\", \"XX00XX00XX00XX00XX000818_XQ01\", \"XX00XX00XX00XX00XX000819_XQ01\", \"XX00XX00XX00XX00XX000820_XQ01\", \"XX00XX00XX00XX00XX000821_XQ01\", \"XX00XX00XX00XX00XX000822_XQ01\", \"XX00XX00XX00XX00XX000823_XQ01\", \"XX00XX00XX00XX00XX000824_XQ01\", \"XX00XX00XX00XX00XX000825_XQ01\", \"XX00XX00XX00XX00XX000826_XQ01\", \"XX00XX00XX00XX00XX000827_XQ01\", \"XX00XX00XX00XX00XX000828_XQ01\", \"XX00XX00XX00XX00XX000829_XQ01\", \"XX00XX00XX00XX00XX000830_XQ01\", \"XX00XX00XX00XX00XX000831_XQ01\", \"XX00XX00XX00XX00XX000832_XQ01\", \"XX00XX00XX00XX00XX000833_XQ01\", \"XX00XX00XX00XX00XX000834_XQ01\", \"XX00XX00XX00XX00XX000835_XQ01\", \"XX00XX00XX00XX00XX000836_XQ01\", \"XX00XX00XX00XX00XX000837_XQ01\", \"XX00XX00XX00XX00XX000838_XQ01\", \"XX00XX00XX00XX00XX000839_XQ01\", \"XX00XX00XX00XX00XX000840_XQ01\", \"XX00XX00XX00XX00XX000841_XQ01\", \"XX00XX00XX00XX00XX000842_XQ01\", \"XX00XX00XX00XX00XX000843_XQ01\", \"XX00XX00XX00XX00XX000844_XQ01\", \"XX00XX00XX00XX00XX000845_XQ01\", \"XX00XX00XX00XX00XX000846_XQ01\", \"XX00XX00XX00XX00XX000847_XQ01\", \"XX00XX00XX00XX00XX000848_XQ01\", \"XX00XX00XX00XX00XX000849_XQ01\", \"XX00XX00XX00XX00XX000850_XQ01\", \"XX00XX00XX00XX00XX000851_XQ01\", \"XX00XX00XX00XX00XX000852_XQ01\", \"XX00XX00XX00XX00XX000853_XQ01\", \"XX00XX00XX00XX00XX000854_XQ01\", \"XX00XX00XX00XX00XX000855_XQ01\", \"XX00XX00XX00XX00XX000856_XQ01\", \"XX00XX00XX00XX00XX000857_XQ01\", \"XX00XX00XX00XX00XX000858_XQ01\", \"XX00XX00XX00XX00XX000859_XQ01\", \"XX00XX00XX00XX00XX000860_XQ01\", \"XX00XX00XX00XX00XX000861_XQ01\", \"XX00XX00XX00XX00XX000862_XQ01\", \"XX00XX00XX00XX00XX000863_XQ01\", \"XX00XX00XX00XX00XX000864_XQ01\", \"XX00XX00XX00XX00XX000865_XQ01\", \"XX00XX00XX00XX00XX000866_XQ01\", \"XX00XX00XX00XX00XX000867_XQ01\", \"XX00XX00XX00XX00XX000868_XQ01\", \"XX00XX00XX00XX00XX000869_XQ01\", \"XX00XX00XX00XX00XX000870_XQ01\", \"XX00XX00XX00XX00XX000871_XQ01\", \"XX00XX00XX00XX00XX000872_XQ01\", \"XX00XX00XX00XX00XX000873_XQ01\", \"XX00XX00XX00XX00XX000874_XQ01\", \"XX00XX00XX00XX00XX000875_XQ01\", \"XX00XX00XX00XX00XX000876_XQ01\", \"XX00XX00XX00XX00XX000877_XQ01\", \"XX00XX00XX00XX00XX000878_XQ01\", \"XX00XX00XX00XX00XX000879_XQ01\", \"XX00XX00XX00XX00XX000880_XQ01\", \"XX00XX00XX00XX00XX000881_XQ01\", \"XX00XX00XX00XX00XX000882_XQ01\", \"XX00XX00XX00XX00XX000883_XQ01\", \"XX00XX00XX00XX00XX000884_XQ01\", \"XX00XX00XX00XX00XX000885_XQ01\", \"XX00XX00XX00XX00XX000886_XQ01\", \"XX00XX00XX00XX00XX000887_XQ01\", \"XX00XX00XX00XX00XX000888_XQ01\", \"XX00XX00XX00XX00XX000889_XQ01\", \"XX00XX00XX00XX00XX000890_XQ01\", \"XX00XX00XX00XX00XX000891_XQ01\", \"XX00XX00XX00XX00XX000892_XQ01\", \"XX00XX00XX00XX00XX000893_XQ01\", \"XX00XX00XX00XX00XX000894_XQ01\", \"XX00XX00XX00XX00XX000895_XQ01\", \"XX00XX00XX00XX00XX000896_XQ01\", \"XX00XX00XX00XX00XX000897_XQ01\", \"XX00XX00XX00XX00XX000898_XQ01\", \"XX00XX00XX00XX00XX000899_XQ01\", \"XX00XX00XX00XX00XX000900_XQ01\", \"XX00XX00XX00XX00XX000901_XQ01\", \"XX00XX00XX00XX00XX000902_XQ01\", \"XX00XX00XX00XX00XX000903_XQ01\", \"XX00XX00XX00XX00XX000904_XQ01\", \"XX00XX00XX00XX00XX000905_XQ01\", \"XX00XX00XX00XX00XX000906_XQ01\", \"XX00XX00XX00XX00XX000907_XQ01\", \"XX00XX00XX00XX00XX000908_XQ01\", \"XX00XX00XX00XX00XX000909_XQ01\", \"XX00XX00XX00XX00XX000910_XQ01\", \"XX00XX00XX00XX00XX000911_XQ01\", \"XX00XX00XX00XX00XX000912_XQ01\", \"XX00XX00XX00XX00XX000913_XQ01\", \"XX00XX00XX00XX00XX000914_XQ01\", \"XX00XX00XX00XX00XX000915_XQ01\", \"XX00XX00XX00XX00XX000916_XQ01\", \"XX00XX00XX00XX00XX000917_XQ01\", \"XX00XX00XX00XX00XX000918_XQ01\", \"XX00XX00XX00XX00XX000919_XQ01\", \"XX00XX00XX00XX00XX000920_XQ01\", \"XX00XX00XX00XX00XX000921_XQ01\", \"XX00XX00XX00XX00XX000922_XQ01\", \"XX00XX00XX00XX00XX000923_XQ01\", \"XX00XX00XX00XX00XX000924_XQ01\", \"XX00XX00XX00XX00XX000925_XQ01\", \"XX00XX00XX00XX00XX000926_XQ01\", \"XX00XX00XX00XX00XX000927_XQ01\", \"XX00XX00XX00XX00XX000928_XQ01\", \"XX00XX00XX00XX00XX000929_XQ01\", \"XX00XX00XX00XX00XX000930_XQ01\", \"XX00XX00XX00XX00XX000931_XQ01\", \"XX00XX00XX00XX00XX000932_XQ01\", \"XX00XX00XX00XX00XX000933_XQ01\", \"XX00XX00XX00XX00XX000934_XQ01\", \"XX00XX00XX00XX00XX000935_XQ01\", \"XX00XX00XX00XX00XX000936_XQ01\", \"XX00XX00XX00XX00XX000937_XQ01\", \"XX00XX00XX00XX00XX000938_XQ01\", \"XX00XX00XX00XX00XX000939_XQ01\", \"XX00XX00XX00XX00XX000940_XQ01\", \"XX00XX00XX00XX00XX000941_XQ01\", \"XX00XX00XX00XX00XX000942_XQ01\", \"XX00XX00XX00XX00XX000943_XQ01\", \"XX00XX00XX00XX00XX000944_XQ01\", \"XX00XX00XX00XX00XX000945_XQ01\", \"XX00XX00XX00XX00XX000946_XQ01\", \"XX00XX00XX00XX00XX000947_XQ01\", \"XX00XX00XX00XX00XX000948_XQ01\", \"XX00XX00XX00XX00XX000949_XQ01\", \"XX00XX00XX00XX00XX000950_XQ01\", \"XX00XX00XX00XX00XX000951_XQ01\", \"XX00XX00XX00XX00XX000952_XQ01\", \"XX00XX00XX00XX00XX000953_XQ01\", \"XX00XX00XX00XX00XX000954_XQ01\", \"XX00XX00XX00XX00XX000955_XQ01\", \"XX00XX00XX00XX00XX000956_XQ01\", \"XX00XX00XX00XX00XX000957_XQ01\", \"XX00XX00XX00XX00XX000958_XQ01\", \"XX00XX00XX00XX00XX000959_XQ01\", \"XX00XX00XX00XX00XX000960_XQ01\", \"XX00XX00XX00XX00XX000961_XQ01\", \"XX00XX00XX00XX00XX000962_XQ01\", \"XX00XX00XX00XX00XX000963_XQ01\", \"XX00XX00XX00XX00XX000964_XQ01\", \"XX00XX00XX00XX00XX000965_XQ01\", \"XX00XX00XX00XX00XX000966_XQ01\", \"XX00XX00XX00XX00XX000967_XQ01\", \"XX00XX00XX00XX00XX000968_XQ01\", \"XX00XX00XX00XX00XX000969_XQ01\", \"XX00XX00XX00XX00XX000970_XQ01\", \"XX00XX00XX00XX00XX000971_XQ01\", \"XX00XX00XX00XX00XX000972_XQ01\", \"XX00XX00XX00XX00XX000973_XQ01\", \"XX00XX00XX00XX00XX000974_XQ01\", \"XX00XX00XX00XX00XX000975_XQ01\", \"XX00XX00XX00XX00XX000976_XQ01\", \"XX00XX00XX00XX00XX000977_XQ01\", \"XX00XX00XX00XX00XX000978_XQ01\", \"XX00XX00XX00XX00XX000979_XQ01\", \"XX00XX00XX00XX00XX000980_XQ01\", \"XX00XX00XX00XX00XX000981_XQ01\", \"XX00XX00XX00XX00XX000982_XQ01\", \"XX00XX00XX00XX00XX000983_XQ01\", \"XX00XX00XX00XX00XX000984_XQ01\", \"XX00XX00XX00XX00XX000985_XQ01\", \"XX00XX00XX00XX00XX000986_XQ01\", \"XX00XX00XX00XX00XX000987_XQ01\", \"XX00XX00XX00XX00XX000988_XQ01\", \"XX00XX00XX00XX00XX000989_XQ01\", \"XX00XX00XX00XX00XX000990_XQ01\", \"XX00XX00XX00XX00XX000991_XQ01\", \"XX00XX00XX00XX00XX000992_XQ01\", \"XX00XX00XX00XX00XX000993_XQ01\", \"XX00XX00XX00XX00XX000994_XQ01\", \"XX00XX00XX00XX00XX000995_XQ01\", \"XX00XX00XX00XX00XX000996_XQ01\", \"XX00XX00XX00XX00XX000997_XQ01\", \"XX00XX00XX00XX00XX000998_XQ01\", \"XX00XX00XX00XX00XX000999_XQ01\", \"XX00XX00XX00XX00XX001000_XQ01\", \"XX00XX00XX00XX00XX001001_XQ01\", \"XX00XX00XX00XX00XX001002_XQ01\", \"XX00XX00XX00XX00XX001003_XQ01\", \"XX00XX00XX00XX00XX001004_XQ01\", \"XX00XX00XX00XX00XX001005_XQ01\", \"XX00XX00XX00XX00XX001006_XQ01\", \"XX00XX00XX00XX00XX001007_XQ01\", \"XX00XX00XX00XX00XX001008_XQ01\", \"XX00XX00XX00XX00XX001009_XQ01\", \"XX00XX00XX00XX00XX001010_XQ01\", \"XX00XX00XX00XX00XX001011_XQ01\", \"XX00XX00XX00XX00XX001012_XQ01\", \"XX00XX00XX00XX00XX001013_XQ01\", \"XX00XX00XX00XX00XX001014_XQ01\", \"XX00XX00XX00XX00XX001015_XQ01\", \"XX00XX00XX00XX00XX001016_XQ01\", \"XX00XX00XX00XX00XX001017_XQ01\", \"XX00XX00XX00XX00XX001018_XQ01\", \"XX00XX00XX00XX00XX001019_XQ01\", \"XX00XX00XX00XX00XX001020_XQ01\", \"XX00XX00XX00XX00XX001021_XQ01\", \"XX00XX00XX00XX00XX001022_XQ01\", \"XX00XX00XX00XX00XX001023_XQ01\", \"XX00XX00XX00XX00XX001024_XQ01\", \"XX00XX00XX00XX00XX001025_XQ01\", \"XX00XX00XX00XX00XX001026_XQ01\", \"XX00XX00XX00XX00XX001027_XQ01\", \"XX00XX00XX00XX00XX001028_XQ01\", \"XX00XX00XX00XX00XX001029_XQ01\", \"XX00XX00XX00XX00XX001030_XQ01\", \"XX00XX00XX00XX00XX001031_XQ01\", \"XX00XX00XX00XX00XX001032_XQ01\", \"XX00XX00XX00XX00XX001033_XQ01\", \"XX00XX00XX00XX00XX001034_XQ01\", \"XX00XX00XX00XX00XX001035_XQ01\", \"XX00XX00XX00XX00XX001036_XQ01\", \"XX00XX00XX00XX00XX001037_XQ01\", \"XX00XX00XX00XX00XX001038_XQ01\", \"XX00XX00XX00XX00XX001039_XQ01\", \"XX00XX00XX00XX00XX001040_XQ01\", \"XX00XX00XX00XX00XX001041_XQ01\", \"XX00XX00XX00XX00XX001042_XQ01\", \"XX00XX00XX00XX00XX001043_XQ01\", \"XX00XX00XX00XX00XX001044_XQ01\", \"XX00XX00XX00XX00XX001045_XQ01\", \"XX00XX00XX00XX00XX001046_XQ01\", \"XX00XX00XX00XX00XX001047_XQ01\", \"XX00XX00XX00XX00XX001048_XQ01\", \"XX00XX00XX00XX00XX001049_XQ01\", \"XX00XX00XX00XX00XX001050_XQ01\", \"XX00XX00XX00XX00XX001051_XQ01\", \"XX00XX00XX00XX00XX001052_XQ01\", \"XX00XX00XX00XX00XX001053_XQ01\", \"XX00XX00XX00XX00XX001054_XQ01\", \"XX00XX00XX00XX00XX001055_XQ01\", \"XX00XX00XX00XX00XX001056_XQ01\", \"XX00XX00XX00XX00XX001057_XQ01\", \"XX00XX00XX00XX00XX001058_XQ01\", \"XX00XX00XX00XX00XX001059_XQ01\", \"XX00XX00XX00XX00XX001060_XQ01\", \"XX00XX00XX00XX00XX001061_XQ01\", \"XX00XX00XX00XX00XX001062_XQ01\", \"XX00XX00XX00XX00XX001063_XQ01\", \"XX00XX00XX00XX00XX001064_XQ01\", \"XX00XX00XX00XX00XX001065_XQ01\", \"XX00XX00XX00XX00XX001066_XQ01\", \"XX00XX00XX00XX00XX001067_XQ01\", \"XX00XX00XX00XX00XX001068_XQ01\", \"XX00XX00XX00XX00XX001069_XQ01\", \"XX00XX00XX00XX00XX001070_XQ01\", \"XX00XX00XX00XX00XX001071_XQ01\", \"XX00XX00XX00XX00XX001072_XQ01\", \"XX00XX00XX00XX00XX001073_XQ01\", \"XX00XX00XX00XX00XX001074_XQ01\", \"XX00XX00XX00XX00XX001075_XQ01\", \"XX00XX00XX00XX00XX001076_XQ01\", \"XX00XX00XX00XX00XX001077_XQ01\", \"XX00XX00XX00XX00XX001078_XQ01\", \"XX00XX00XX00XX00XX001079_XQ01\", \"XX00XX00XX00XX00XX001080_XQ01\", \"XX00XX00XX00XX00XX001081_XQ01\", \"XX00XX00XX00XX00XX001082_XQ01\", \"XX00XX00XX00XX00XX001083_XQ01\", \"XX00XX00XX00XX00XX001084_XQ01\", \"XX00XX00XX00XX00XX001085_XQ01\", \"XX00XX00XX00XX00XX001086_XQ01\", \"XX00XX00XX00XX00XX001087_XQ01\", \"XX00XX00XX00XX00XX001088_XQ01\", \"XX00XX00XX00XX00XX001089_XQ01\", \"XX00XX00XX00XX00XX001090_XQ01\", \"XX00XX00XX00XX00XX001091_XQ01\", \"XX00XX00XX00XX00XX001092_XQ01\", \"XX00XX00XX00XX00XX001093_XQ01\", \"XX00XX00XX00XX00XX001094_XQ01\", \"XX00XX00XX00XX00XX001095_XQ01\", \"XX00XX00XX00XX00XX001096_XQ01\", \"XX00XX00XX00XX00XX001097_XQ01\", \"XX00XX00XX00XX00XX001098_XQ01\", \"XX00XX00XX00XX00XX001099_XQ01\", \"XX00XX00XX00XX00XX001100_XQ01\", \"XX00XX00XX00XX00XX001101_XQ01\", \"XX00XX00XX00XX00XX001102_XQ01\", \"XX00XX00XX00XX00XX001103_XQ01\", \"XX00XX00XX00XX00XX001104_XQ01\", \"XX00XX00XX00XX00XX001105_XQ01\", \"XX00XX00XX00XX00XX001106_XQ01\", \"XX00XX00XX00XX00XX001107_XQ01\", \"XX00XX00XX00XX00XX001108_XQ01\", \"XX00XX00XX00XX00XX001109_XQ01\", \"XX00XX00XX00XX00XX001110_XQ01\", \"XX00XX00XX00XX00XX001111_XQ01\", \"XX00XX00XX00XX00XX001112_XQ01\", \"XX00XX00XX00XX00XX001113_XQ01\", \"XX00XX00XX00XX00XX001114_XQ01\", \"XX00XX00XX00XX00XX001115_XQ01\", \"XX00XX00XX00XX00XX001116_XQ01\", \"XX00XX00XX00XX00XX001117_XQ01\", \"XX00XX00XX00XX00XX001118_XQ01\", \"XX00XX00XX00XX00XX001119_XQ01\", \"XX00XX00XX00XX00XX001120_XQ01\", \"XX00XX00XX00XX00XX001121_XQ01\", \"XX00XX00XX00XX00XX001122_XQ01\", \"XX00XX00XX00XX00XX001123_XQ01\", \"XX00XX00XX00XX00XX001124_XQ01\", \"XX00XX00XX00XX00XX001125_XQ01\", \"XX00XX00XX00XX00XX001126_XQ01\", \"XX00XX00XX00XX00XX001127_XQ01\", \"XX00XX00XX00XX00XX001128_XQ01\", \"XX00XX00XX00XX00XX001129_XQ01\", \"XX00XX00XX00XX00XX001130_XQ01\", \"XX00XX00XX00XX00XX001131_XQ01\", \"XX00XX00XX00XX00XX001132_XQ01\", \"XX00XX00XX00XX00XX001133_XQ01\", \"XX00XX00XX00XX00XX001134_XQ01\", \"XX00XX00XX00XX00XX001135_XQ01\", \"XX00XX00XX00XX00XX001136_XQ01\", \"XX00XX00XX00XX00XX001137_XQ01\", \"XX00XX00XX00XX00XX001138_XQ01\", \"XX00XX00XX00XX00XX001139_XQ01\", \"XX00XX00XX00XX00XX001140_XQ01\", \"XX00XX00XX00XX00XX001141_XQ01\", \"XX00XX00XX00XX00XX001142_XQ01\", \"XX00XX00XX00XX00XX001143_XQ01\", \"XX00XX00XX00XX00XX001144_XQ01\", \"XX00XX00XX00XX00XX001145_XQ01\", \"XX00XX00XX00XX00XX001146_XQ01\", \"XX00XX00XX00XX00XX001147_XQ01\", \"XX00XX00XX00XX00XX001148_XQ01\", \"XX00XX00XX00XX00XX001149_XQ01\", \"XX00XX00XX00XX00XX001150_XQ01\", \"XX00XX00XX00XX00XX001151_XQ01\", \"XX00XX00XX00XX00XX001152_XQ01\", \"XX00XX00XX00XX00XX001153_XQ01\", \"XX00XX00XX00XX00XX001154_XQ01\", \"XX00XX00XX00XX00XX001155_XQ01\", \"XX00XX00XX00XX00XX001156_XQ01\", \"XX00XX00XX00XX00XX001157_XQ01\", \"XX00XX00XX00XX00XX001158_XQ01\", \"XX00XX00XX00XX00XX001159_XQ01\", \"XX00XX00XX00XX00XX001160_XQ01\", \"XX00XX00XX00XX00XX001161_XQ01\", \"XX00XX00XX00XX00XX001162_XQ01\", \"XX00XX00XX00XX00XX001163_XQ01\", \"XX00XX00XX00XX00XX001164_XQ01\", \"XX00XX00XX00XX00XX001165_XQ01\", \"XX00XX00XX00XX00XX001166_XQ01\", \"XX00XX00XX00XX00XX001167_XQ01\", \"XX00XX00XX00XX00XX001168_XQ01\", \"XX00XX00XX00XX00XX001169_XQ01\", \"XX00XX00XX00XX00XX001170_XQ01\", \"XX00XX00XX00XX00XX001171_XQ01\", \"XX00XX00XX00XX00XX001172_XQ01\", \"XX00XX00XX00XX00XX001173_XQ01\", \"XX00XX00XX00XX00XX001174_XQ01\", \"XX00XX00XX00XX00XX001175_XQ01\", \"XX00XX00XX00XX00XX001176_XQ01\", \"XX00XX00XX00XX00XX001177_XQ01\", \"XX00XX00XX00XX00XX001178_XQ01\", \"XX00XX00XX00XX00XX001179_XQ01\", \"XX00XX00XX00XX00XX001180_XQ01\", \"XX00XX00XX00XX00XX001181_XQ01\", \"XX00XX00XX00XX00XX001182_XQ01\", \"XX00XX00XX00XX00XX001183_XQ01\", \"XX00XX00XX00XX00XX001184_XQ01\", \"XX00XX00XX00XX00XX001185_XQ01\", \"XX00XX00XX00XX00XX001186_XQ01\", \"XX00XX00XX00XX00XX001187_XQ01\", \"XX00XX00XX00XX00XX001188_XQ01\", \"XX00XX00XX00XX00XX001189_XQ01\", \"XX00XX00XX00XX00XX001190_XQ01\", \"XX00XX00XX00XX00XX001191_XQ01\", \"XX00XX00XX00XX00XX001192_XQ01\", \"XX00XX00XX00XX00XX001193_XQ01\", \"XX00XX00XX00XX00XX001194_XQ01\", \"XX00XX00XX00XX00XX001195_XQ01\", \"XX00XX00XX00XX00XX001196_XQ01\", \"XX00XX00XX00XX00XX001197_XQ01\", \"XX00XX00XX00XX00XX001198_XQ01\", \"XX00XX00XX00XX00XX001199_XQ01\", \"XX00XX00XX00XX00XX001200_XQ01\", \"XX00XX00XX00XX00XX001201_XQ01\", \"XX00XX00XX00XX00XX001202_XQ01\", \"XX00XX00XX00XX00XX001203_XQ01\", \"XX00XX00XX00XX00XX001204_XQ01\", \"XX00XX00XX00XX00XX001205_XQ01\", \"XX00XX00XX00XX00XX001206_XQ01\", \"XX00XX00XX00XX00XX001207_XQ01\", \"XX00XX00XX00XX00XX001208_XQ01\", \"XX00XX00XX00XX00XX001209_XQ01\", \"XX00XX00XX00XX00XX001210_XQ01\", \"XX00XX00XX00XX00XX001211_XQ01\", \"XX00XX00XX00XX00XX001212_XQ01\", \"XX00XX00XX00XX00XX001213_XQ01\", \"XX00XX00XX00XX00XX001214_XQ01\", \"XX00XX00XX00XX00XX001215_XQ01\", \"XX00XX00XX00XX00XX001216_XQ01\", \"XX00XX00XX00XX00XX001217_XQ01\", \"XX00XX00XX00XX00XX001218_XQ01\", \"XX00XX00XX00XX00XX001219_XQ01\", \"XX00XX00XX00XX00XX001220_XQ01\", \"XX00XX00XX00XX00XX001221_XQ01\", \"XX00XX00XX00XX00XX001222_XQ01\", \"XX00XX00XX00XX00XX001223_XQ01\", \"XX00XX00XX00XX00XX001224_XQ01\", \"XX00XX00XX00XX00XX001225_XQ01\", \"XX00XX00XX00XX00XX001226_XQ01\", \"XX00XX00XX00XX00XX001227_XQ01\", \"XX00XX00XX00XX00XX001228_XQ01\", \"XX00XX00XX00XX00XX001229_XQ01\", \"XX00XX00XX00XX00XX001230_XQ01\", \"XX00XX00XX00XX00XX001231_XQ01\", \"XX00XX00XX00XX00XX001232_XQ01\", \"XX00XX00XX00XX00XX001233_XQ01\", \"XX00XX00XX00XX00XX001234_XQ01\", \"XX00XX00XX00XX00XX001235_XQ01\", \"XX00XX00XX00XX00XX001236_XQ01\", \"XX00XX00XX00XX00XX001237_XQ01\", \"XX00XX00XX00XX00XX001238_XQ01\", \"XX00XX00XX00XX00XX001239_XQ01\", \"XX00XX00XX00XX00XX001240_XQ01\", \"XX00XX00XX00XX00XX001241_XQ01\", \"XX00XX00XX00XX00XX001242_XQ01\", \"XX00XX00XX00XX00XX001243_XQ01\", \"XX00XX00XX00XX00XX001244_XQ01\", \"XX00XX00XX00XX00XX001245_XQ01\", \"XX00XX00XX00XX00XX001246_XQ01\", \"XX00XX00XX00XX00XX001247_XQ01\", \"XX00XX00XX00XX00XX001248_XQ01\", \"XX00XX00XX00XX00XX001249_XQ01\", \"XX00XX00XX00XX00XX001250_XQ01\", \"XX00XX00XX00XX00XX001251_XQ01\", \"XX00XX00XX00XX00XX001252_XQ01\", \"XX00XX00XX00XX00XX001253_XQ01\", \"XX00XX00XX00XX00XX001254_XQ01\", \"XX00XX00XX00XX00XX001255_XQ01\", \"XX00XX00XX00XX00XX001256_XQ01\", \"XX00XX00XX00XX00XX001257_XQ01\", \"XX00XX00XX00XX00XX001258_XQ01\", \"XX00XX00XX00XX00XX001259_XQ01\", \"XX00XX00XX00XX00XX001260_XQ01\", \"XX00XX00XX00XX00XX001261_XQ01\", \"XX00XX00XX00XX00XX001262_XQ01\", \"XX00XX00XX00XX00XX001263_XQ01\", \"XX00XX00XX00XX00XX001264_XQ01\", \"XX00XX00XX00XX00XX001265_XQ01\", \"XX00XX00XX00XX00XX001266_XQ01\", \"XX00XX00XX00XX00XX001267_XQ01\", \"XX00XX00XX00XX00XX001268_XQ01\", \"XX00XX00XX00XX00XX001269_XQ01\", \"XX00XX00XX00XX00XX001270_XQ01\", \"XX00XX00XX00XX00XX001271_XQ01\", \"XX00XX00XX00XX00XX001272_XQ01\", \"XX00XX00XX00XX00XX001273_XQ01\", \"XX00XX00XX00XX00XX001274_XQ01\", \"XX00XX00XX00XX00XX001275_XQ01\", \"XX00XX00XX00XX00XX001276_XQ01\", \"XX00XX00XX00XX00XX001277_XQ01\", \"XX00XX00XX00XX00XX001278_XQ01\", \"XX00XX00XX00XX00XX001279_XQ01\", \"XX00XX00XX00XX00XX001280_XQ01\", \"XX00XX00XX00XX00XX001281_XQ01\", \"XX00XX00XX00XX00XX001282_XQ01\", \"XX00XX00XX00XX00XX001283_XQ01\", \"XX00XX00XX00XX00XX001284_XQ01\", \"XX00XX00XX00XX00XX001285_XQ01\", \"XX00XX00XX00XX00XX001286_XQ01\", \"XX00XX00XX00XX00XX001287_XQ01\", \"XX00XX00XX00XX00XX001288_XQ01\", \"XX00XX00XX00XX00XX001289_XQ01\", \"XX00XX00XX00XX00XX001290_XQ01\", \"XX00XX00XX00XX00XX001291_XQ01\", \"XX00XX00XX00XX00XX001292_XQ01\", \"XX00XX00XX00XX00XX001293_XQ01\", \"XX00XX00XX00XX00XX001294_XQ01\", \"XX00XX00XX00XX00XX001295_XQ01\", \"XX00XX00XX00XX00XX001296_XQ01\", \"XX00XX00XX00XX00XX001297_XQ01\", \"XX00XX00XX00XX00XX001298_XQ01\", \"XX00XX00XX00XX00XX001299_XQ01\", \"XX00XX00XX00XX00XX001300_XQ01\", \"XX00XX00XX00XX00XX001301_XQ01\", \"XX00XX00XX00XX00XX001302_XQ01\", \"XX00XX00XX00XX00XX001303_XQ01\", \"XX00XX00XX00XX00XX001304_XQ01\", \"XX00XX00XX00XX00XX001305_XQ01\", \"XX00XX00XX00XX00XX001306_XQ01\", \"XX00XX00XX00XX00XX001307_XQ01\", \"XX00XX00XX00XX00XX001308_XQ01\", \"XX00XX00XX00XX00XX001309_XQ01\", \"XX00XX00XX00XX00XX001310_XQ01\", \"XX00XX00XX00XX00XX001311_XQ01\", \"XX00XX00XX00XX00XX001312_XQ01\", \"XX00XX00XX00XX00XX001313_XQ01\", \"XX00XX00XX00XX00XX001314_XQ01\", \"XX00XX00XX00XX00XX001315_XQ01\", \"XX00XX00XX00XX00XX001316_XQ01\", \"XX00XX00XX00XX00XX001317_XQ01\", \"XX00XX00XX00XX00XX001318_XQ01\", \"XX00XX00XX00XX00XX001319_XQ01\", \"XX00XX00XX00XX00XX001320_XQ01\", \"XX00XX00XX00XX00XX001321_XQ01\", \"XX00XX00XX00XX00XX001322_XQ01\", \"XX00XX00XX00XX00XX001323_XQ01\", \"XX00XX00XX00XX00XX001324_XQ01\", \"XX00XX00XX00XX00XX001325_XQ01\", \"XX00XX00XX00XX00XX001326_XQ01\", \"XX00XX00XX00XX00XX001327_XQ01\", \"XX00XX00XX00XX00XX001328_XQ01\", \"XX00XX00XX00XX00XX001329_XQ01\", \"XX00XX00XX00XX00XX001330_XQ01\", \"XX00XX00XX00XX00XX001331_XQ01\", \"XX00XX00XX00XX00XX001332_XQ01\", \"XX00XX00XX00XX00XX001333_XQ01\", \"XX00XX00XX00XX00XX001334_XQ01\", \"XX00XX00XX00XX00XX001335_XQ01\", \"XX00XX00XX00XX00XX001336_XQ01\", \"XX00XX00XX00XX00XX001337_XQ01\", \"XX00XX00XX00XX00XX001338_XQ01\", \"XX00XX00XX00XX00XX001339_XQ01\", \"XX00XX00XX00XX00XX001340_XQ01\", \"XX00XX00XX00XX00XX001341_XQ01\", \"XX00XX00XX00XX00XX001342_XQ01\", \"XX00XX00XX00XX00XX001343_XQ01\", \"XX00XX00XX00XX00XX001344_XQ01\", \"XX00XX00XX00XX00XX001345_XQ01\", \"XX00XX00XX00XX00XX001346_XQ01\", \"XX00XX00XX00XX00XX001347_XQ01\", \"XX00XX00XX00XX00XX001348_XQ01\", \"XX00XX00XX00XX00XX001349_XQ01\", \"XX00XX00XX00XX00XX001350_XQ01\", \"XX00XX00XX00XX00XX001351_XQ01\", \"XX00XX00XX00XX00XX001352_XQ01\", \"XX00XX00XX00XX00XX001353_XQ01\", \"XX00XX00XX00XX00XX001354_XQ01\", \"XX00XX00XX00XX00XX001355_XQ01\", \"XX00XX00XX00XX00XX001356_XQ01\", \"XX00XX00XX00XX00XX001357_XQ01\", \"XX00XX00XX00XX00XX001358_XQ01\", \"XX00XX00XX00XX00XX001359_XQ01\", \"XX00XX00XX00XX00XX001360_XQ01\", \"XX00XX00XX00XX00XX001361_XQ01\", \"XX00XX00XX00XX00XX001362_XQ01\", \"XX00XX00XX00XX00XX001363_XQ01\", \"XX00XX00XX00XX00XX001364_XQ01\", \"XX00XX00XX00XX00XX001365_XQ01\", \"XX00XX00XX00XX00XX001366_XQ01\", \"XX00XX00XX00XX00XX001367_XQ01\", \"XX00XX00XX00XX00XX001368_XQ01\", \"XX00XX00XX00XX00XX001369_XQ01\", \"XX00XX00XX00XX00XX001370_XQ01\", \"XX00XX00XX00XX00XX001371_XQ01\", \"XX00XX00XX00XX00XX001372_XQ01\", \"XX00XX00XX00XX00XX001373_XQ01\", \"XX00XX00XX00XX00XX001374_XQ01\", \"XX00XX00XX00XX00XX001375_XQ01\", \"XX00XX00XX00XX00XX001376_XQ01\", \"XX00XX00XX00XX00XX001377_XQ01\", \"XX00XX00XX00XX00XX001378_XQ01\", \"XX00XX00XX00XX00XX001379_XQ01\", \"XX00XX00XX00XX00XX001380_XQ01\", \"XX00XX00XX00XX00XX001381_XQ01\", \"XX00XX00XX00XX00XX001382_XQ01\", \"XX00XX00XX00XX00XX001383_XQ01\", \"XX00XX00XX00XX00XX001384_XQ01\", \"XX00XX00XX00XX00XX001385_XQ01\", \"XX00XX00XX00XX00XX001386_XQ01\", \"XX00XX00XX00XX00XX001387_XQ01\", \"XX00XX00XX00XX00XX001388_XQ01\", \"XX00XX00XX00XX00XX001389_XQ01\", \"XX00XX00XX00XX00XX001390_XQ01\", \"XX00XX00XX00XX00XX001391_XQ01\", \"XX00XX00XX00XX00XX001392_XQ01\", \"XX00XX00XX00XX00XX001393_XQ01\", \"XX00XX00XX00XX00XX001394_XQ01\", \"XX00XX00XX00XX00XX001395_XQ01\", \"XX00XX00XX00XX00XX001396_XQ01\", \"XX00XX00XX00XX00XX001397_XQ01\", \"XX00XX00XX00XX00XX001398_XQ01\", \"XX00XX00XX00XX00XX001399_XQ01\", \"XX00XX00XX00XX00XX001400_XQ01\", \"XX00XX00XX00XX00XX001401_XQ01\", \"XX00XX00XX00XX00XX001402_XQ01\", \"XX00XX00XX00XX00XX001403_XQ01\", \"XX00XX00XX00XX00XX001404_XQ01\", \"XX00XX00XX00XX00XX001405_XQ01\", \"XX00XX00XX00XX00XX001406_XQ01\", \"XX00XX00XX00XX00XX001407_XQ01\", \"XX00XX00XX00XX00XX001408_XQ01\", \"XX00XX00XX00XX00XX001409_XQ01\", \"XX00XX00XX00XX00XX001410_XQ01\", \"XX00XX00XX00XX00XX001411_XQ01\", \"XX00XX00XX00XX00XX001412_XQ01\", \"XX00XX00XX00XX00XX001413_XQ01\", \"XX00XX00XX00XX00XX001414_XQ01\", \"XX00XX00XX00XX00XX001415_XQ01\", \"XX00XX00XX00XX00XX001416_XQ01\", \"XX00XX00XX00XX00XX001417_XQ01\", \"XX00XX00XX00XX00XX001418_XQ01\", \"XX00XX00XX00XX00XX001419_XQ01\", \"XX00XX00XX00XX00XX001420_XQ01\", \"XX00XX00XX00XX00XX001421_XQ01\", \"XX00XX00XX00XX00XX001422_XQ01\", \"XX00XX00XX00XX00XX001423_XQ01\", \"XX00XX00XX00XX00XX001424_XQ01\", \"XX00XX00XX00XX00XX001425_XQ01\", \"XX00XX00XX00XX00XX001426_XQ01\", \"XX00XX00XX00XX00XX001427_XQ01\", \"XX00XX00XX00XX00XX001428_XQ01\", \"XX00XX00XX00XX00XX001429_XQ01\", \"XX00XX00XX00XX00XX001430_XQ01\", \"XX00XX00XX00XX00XX001431_XQ01\", \"XX00XX00XX00XX00XX001432_XQ01\", \"XX00XX00XX00XX00XX001433_XQ01\", \"XX00XX00XX00XX00XX001434_XQ01\", \"XX00XX00XX00XX00XX001435_XQ01\", \"XX00XX00XX00XX00XX001436_XQ01\", \"XX00XX00XX00XX00XX001437_XQ01\", \"XX00XX00XX00XX00XX001438_XQ01\", \"XX00XX00XX00XX00XX001439_XQ01\", \"XX00XX00XX00XX00XX001440_XQ01\", \"XX00XX00XX00XX00XX001441_XQ01\", \"XX00XX00XX00XX00XX001442_XQ01\", \"XX00XX00XX00XX00XX001443_XQ01\", \"XX00XX00XX00XX00XX001444_XQ01\", \"XX00XX00XX00XX00XX001445_XQ01\", \"XX00XX00XX00XX00XX001446_XQ01\", \"XX00XX00XX00XX00XX001447_XQ01\", \"XX00XX00XX00XX00XX001448_XQ01\", \"XX00XX00XX00XX00XX001449_XQ01\", \"XX00XX00XX00XX00XX001450_XQ01\", \"XX00XX00XX00XX00XX001451_XQ01\", \"XX00XX00XX00XX00XX001452_XQ01\", \"XX00XX00XX00XX00XX001453_XQ01\", \"XX00XX00XX00XX00XX001454_XQ01\", \"XX00XX00XX00XX00XX001455_XQ01\", \"XX00XX00XX00XX00XX001456_XQ01\", \"XX00XX00XX00XX00XX001457_XQ01\", \"XX00XX00XX00XX00XX001458_XQ01\", \"XX00XX00XX00XX00XX001459_XQ01\", \"XX00XX00XX00XX00XX001460_XQ01\", \"XX00XX00XX00XX00XX001461_XQ01\", \"XX00XX00XX00XX00XX001462_XQ01\", \"XX00XX00XX00XX00XX001463_XQ01\", \"XX00XX00XX00XX00XX001464_XQ01\", \"XX00XX00XX00XX00XX001465_XQ01\", \"XX00XX00XX00XX00XX001466_XQ01\", \"XX00XX00XX00XX00XX001467_XQ01\", \"XX00XX00XX00XX00XX001468_XQ01\", \"XX00XX00XX00XX00XX001469_XQ01\", \"XX00XX00XX00XX00XX001470_XQ01\", \"XX00XX00XX00XX00XX001471_XQ01\", \"XX00XX00XX00XX00XX001472_XQ01\", \"XX00XX00XX00XX00XX001473_XQ01\", \"XX00XX00XX00XX00XX001474_XQ01\", \"XX00XX00XX00XX00XX001475_XQ01\", \"XX00XX00XX00XX00XX001476_XQ01\", \"XX00XX00XX00XX00XX001477_XQ01\", \"XX00XX00XX00XX00XX001478_XQ01\", \"XX00XX00XX00XX00XX001479_XQ01\", \"XX00XX00XX00XX00XX001480_XQ01\", \"XX00XX00XX00XX00XX001481_XQ01\", \"XX00XX00XX00XX00XX001482_XQ01\", \"XX00XX00XX00XX00XX001483_XQ01\", \"XX00XX00XX00XX00XX001484_XQ01\", \"XX00XX00XX00XX00XX001485_XQ01\", \"XX00XX00XX00XX00XX001486_XQ01\", \"XX00XX00XX00XX00XX001487_XQ01\", \"XX00XX00XX00XX00XX001488_XQ01\", \"XX00XX00XX00XX00XX001489_XQ01\", \"XX00XX00XX00XX00XX001490_XQ01\", \"XX00XX00XX00XX00XX001491_XQ01\", \"XX00XX00XX00XX00XX001492_XQ01\", \"XX00XX00XX00XX00XX001493_XQ01\", \"XX00XX00XX00XX00XX001494_XQ01\", \"XX00XX00XX00XX00XX001495_XQ01\", \"XX00XX00XX00XX00XX001496_XQ01\", \"XX00XX00XX00XX00XX001497_XQ01\", \"XX00XX00XX00XX00XX001498_XQ01\", \"XX00XX00XX00XX00XX001499_XQ01\") \nVALUES ( '2017-11-07 12:04:06.000', 0.00000E+0, 1.00000E+0, 2.00000E+0, 3.00000E+0, 4.00000E+0, 5.00000E+0, 6.00000E+0, 7.00000E+0, 8.00000E+0, 9.00000E+0, 1.00000E+1, 1.10000E+1, 1.20000E+1, 1.30000E+1, 1.40000E+1, 1.50000E+1, 1.60000E+1, 1.70000E+1, 1.80000E+1, 1.90000E+1, 2.00000E+1, 2.10000E+1, 2.20000E+1, 2.30000E+1, 2.40000E+1, 2.50000E+1, 2.60000E+1, 2.70000E+1, 2.80000E+1, 2.90000E+1, 3.00000E+1, 3.10000E+1, 3.20000E+1, 3.30000E+1, 3.40000E+1, 3.50000E+1, 3.60000E+1, 3.70000E+1, 3.80000E+1, 3.90000E+1, 4.00000E+1, 4.10000E+1, 4.20000E+1, 4.30000E+1, 4.40000E+1, 4.50000E+1, 4.60000E+1, 4.70000E+1, 4.80000E+1, 4.90000E+1, 5.00000E+1, 5.10000E+1, 5.20000E+1, 5.30000E+1, 5.40000E+1, 5.50000E+1, 5.60000E+1, 5.70000E+1, 5.80000E+1, 5.90000E+1, 6.00000E+1, 6.10000E+1, 6.20000E+1, 6.30000E+1, 6.40000E+1, 6.50000E+1, 6.60000E+1, 6.70000E+1, 6.80000E+1, 6.90000E+1, 7.00000E+1, 7.10000E+1, 7.20000E+1, 7.30000E+1, 7.40000E+1, 7.50000E+1, 7.60000E+1, 7.70000E+1, 7.80000E+1, 7.90000E+1, 8.00000E+1, 8.10000E+1, 8.20000E+1, 8.30000E+1, 8.40000E+1, 8.50000E+1, 8.60000E+1, 8.70000E+1, 8.80000E+1, 8.90000E+1, 9.00000E+1, 9.10000E+1, 9.20000E+1, 9.30000E+1, 9.40000E+1, 9.50000E+1, 9.60000E+1, 9.70000E+1, 9.80000E+1, 9.90000E+1, 1.00000E+2, 1.01000E+2, 1.02000E+2, 1.03000E+2, 1.04000E+2, 1.05000E+2, 1.06000E+2, 1.07000E+2, 1.08000E+2, 1.09000E+2, 1.10000E+2, 1.11000E+2, 1.12000E+2, 1.13000E+2, 1.14000E+2, 1.15000E+2, 1.16000E+2, 1.17000E+2, 1.18000E+2, 1.19000E+2, 1.20000E+2, 1.21000E+2, 1.22000E+2, 1.23000E+2, 1.24000E+2, 1.25000E+2, 1.26000E+2, 1.27000E+2, 1.28000E+2, 1.29000E+2, 1.30000E+2, 1.31000E+2, 1.32000E+2, 1.33000E+2, 1.34000E+2, 1.35000E+2, 1.36000E+2, 1.37000E+2, 1.38000E+2, 1.39000E+2, 1.40000E+2, 1.41000E+2, 1.42000E+2, 1.43000E+2, 1.44000E+2, 1.45000E+2, 1.46000E+2, 1.47000E+2, 1.48000E+2, 1.49000E+2, 1.50000E+2, 1.51000E+2, 1.52000E+2, 1.53000E+2, 1.54000E+2, 1.55000E+2, 1.56000E+2, 1.57000E+2, 1.58000E+2, 1.59000E+2, 1.60000E+2, 1.61000E+2, 1.62000E+2, 1.63000E+2, 1.64000E+2, 1.65000E+2, 1.66000E+2, 1.67000E+2, 1.68000E+2, 1.69000E+2, 1.70000E+2, 1.71000E+2, 1.72000E+2, 1.73000E+2, 1.74000E+2, 1.75000E+2, 1.76000E+2, 1.77000E+2, 1.78000E+2, 1.79000E+2, 1.80000E+2, 1.81000E+2, 1.82000E+2, 1.83000E+2, 1.84000E+2, 1.85000E+2, 1.86000E+2, 1.87000E+2, 1.88000E+2, 1.89000E+2, 1.90000E+2, 1.91000E+2, 1.92000E+2, 1.93000E+2, 1.94000E+2, 1.95000E+2, 1.96000E+2, 1.97000E+2, 1.98000E+2, 1.99000E+2, 2.00000E+2, 2.01000E+2, 2.02000E+2, 2.03000E+2, 2.04000E+2, 2.05000E+2, 2.06000E+2, 2.07000E+2, 2.08000E+2, 2.09000E+2, 2.10000E+2, 2.11000E+2, 2.12000E+2, 2.13000E+2, 2.14000E+2, 2.15000E+2, 2.16000E+2, 2.17000E+2, 2.18000E+2, 2.19000E+2, 2.20000E+2, 2.21000E+2, 2.22000E+2, 2.23000E+2, 2.24000E+2, 2.25000E+2, 2.26000E+2, 2.27000E+2, 2.28000E+2, 2.29000E+2, 2.30000E+2, 2.31000E+2, 2.32000E+2, 2.33000E+2, 2.34000E+2, 2.35000E+2, 2.36000E+2, 2.37000E+2, 2.38000E+2, 2.39000E+2, 2.40000E+2, 2.41000E+2, 2.42000E+2, 2.43000E+2, 2.44000E+2, 2.45000E+2, 2.46000E+2, 2.47000E+2, 2.48000E+2, 2.49000E+2, 2.50000E+2, 2.51000E+2, 2.52000E+2, 2.53000E+2, 2.54000E+2, 2.55000E+2, 2.56000E+2, 2.57000E+2, 2.58000E+2, 2.59000E+2, 2.60000E+2, 2.61000E+2, 2.62000E+2, 2.63000E+2, 2.64000E+2, 2.65000E+2, 2.66000E+2, 2.67000E+2, 2.68000E+2, 2.69000E+2, 2.70000E+2, 2.71000E+2, 2.72000E+2, 2.73000E+2, 2.74000E+2, 2.75000E+2, 2.76000E+2, 2.77000E+2, 2.78000E+2, 2.79000E+2, 2.80000E+2, 2.81000E+2, 2.82000E+2, 2.83000E+2, 2.84000E+2, 2.85000E+2, 2.86000E+2, 2.87000E+2, 2.88000E+2, 2.89000E+2, 2.90000E+2, 2.91000E+2, 2.92000E+2, 2.93000E+2, 2.94000E+2, 2.95000E+2, 2.96000E+2, 2.97000E+2, 2.98000E+2, 2.99000E+2, 3.00000E+2, 3.01000E+2, 3.02000E+2, 3.03000E+2, 3.04000E+2, 3.05000E+2, 3.06000E+2, 3.07000E+2, 3.08000E+2, 3.09000E+2, 3.10000E+2, 3.11000E+2, 3.12000E+2, 3.13000E+2, 3.14000E+2, 3.15000E+2, 3.16000E+2, 3.17000E+2, 3.18000E+2, 3.19000E+2, 3.20000E+2, 3.21000E+2, 3.22000E+2, 3.23000E+2, 3.24000E+2, 3.25000E+2, 3.26000E+2, 3.27000E+2, 3.28000E+2, 3.29000E+2, 3.30000E+2, 3.31000E+2, 3.32000E+2, 3.33000E+2, 3.34000E+2, 3.35000E+2, 3.36000E+2, 3.37000E+2, 3.38000E+2, 3.39000E+2, 3.40000E+2, 3.41000E+2, 3.42000E+2, 3.43000E+2, 3.44000E+2, 3.45000E+2, 3.46000E+2, 3.47000E+2, 3.48000E+2, 3.49000E+2, 3.50000E+2, 3.51000E+2, 3.52000E+2, 3.53000E+2, 3.54000E+2, 3.55000E+2, 3.56000E+2, 3.57000E+2, 3.58000E+2, 3.59000E+2, 3.60000E+2, 3.61000E+2, 3.62000E+2, 3.63000E+2, 3.64000E+2, 3.65000E+2, 3.66000E+2, 3.67000E+2, 3.68000E+2, 3.69000E+2, 3.70000E+2, 3.71000E+2, 3.72000E+2, 3.73000E+2, 3.74000E+2, 3.75000E+2, 3.76000E+2, 3.77000E+2, 3.78000E+2, 3.79000E+2, 3.80000E+2, 3.81000E+2, 3.82000E+2, 3.83000E+2, 3.84000E+2, 3.85000E+2, 3.86000E+2, 3.87000E+2, 3.88000E+2, 3.89000E+2, 3.90000E+2, 3.91000E+2, 3.92000E+2, 3.93000E+2, 3.94000E+2, 3.95000E+2, 3.96000E+2, 3.97000E+2, 3.98000E+2, 3.99000E+2, 4.00000E+2, 4.01000E+2, 4.02000E+2, 4.03000E+2, 4.04000E+2, 4.05000E+2, 4.06000E+2, 4.07000E+2, 4.08000E+2, 4.09000E+2, 4.10000E+2, 4.11000E+2, 4.12000E+2, 4.13000E+2, 4.14000E+2, 4.15000E+2, 4.16000E+2, 4.17000E+2, 4.18000E+2, 4.19000E+2, 4.20000E+2, 4.21000E+2, 4.22000E+2, 4.23000E+2, 4.24000E+2, 4.25000E+2, 4.26000E+2, 4.27000E+2, 4.28000E+2, 4.29000E+2, 4.30000E+2, 4.31000E+2, 4.32000E+2, 4.33000E+2, 4.34000E+2, 4.35000E+2, 4.36000E+2, 4.37000E+2, 4.38000E+2, 4.39000E+2, 4.40000E+2, 4.41000E+2, 4.42000E+2, 4.43000E+2, 4.44000E+2, 4.45000E+2, 4.46000E+2, 4.47000E+2, 4.48000E+2, 4.49000E+2, 4.50000E+2, 4.51000E+2, 4.52000E+2, 4.53000E+2, 4.54000E+2, 4.55000E+2, 4.56000E+2, 4.57000E+2, 4.58000E+2, 4.59000E+2, 4.60000E+2, 4.61000E+2, 4.62000E+2, 4.63000E+2, 4.64000E+2, 4.65000E+2, 4.66000E+2, 4.67000E+2, 4.68000E+2, 4.69000E+2, 4.70000E+2, 4.71000E+2, 4.72000E+2, 4.73000E+2, 4.74000E+2, 4.75000E+2, 4.76000E+2, 4.77000E+2, 4.78000E+2, 4.79000E+2, 4.80000E+2, 4.81000E+2, 4.82000E+2, 4.83000E+2, 4.84000E+2, 4.85000E+2, 4.86000E+2, 4.87000E+2, 4.88000E+2, 4.89000E+2, 4.90000E+2, 4.91000E+2, 4.92000E+2, 4.93000E+2, 4.94000E+2, 4.95000E+2, 4.96000E+2, 4.97000E+2, 4.98000E+2, 4.99000E+2, 5.00000E+2, 5.01000E+2, 5.02000E+2, 5.03000E+2, 5.04000E+2, 5.05000E+2, 5.06000E+2, 5.07000E+2, 5.08000E+2, 5.09000E+2, 5.10000E+2, 5.11000E+2, 5.12000E+2, 5.13000E+2, 5.14000E+2, 5.15000E+2, 5.16000E+2, 5.17000E+2, 5.18000E+2, 5.19000E+2, 5.20000E+2, 5.21000E+2, 5.22000E+2, 5.23000E+2, 5.24000E+2, 5.25000E+2, 5.26000E+2, 5.27000E+2, 5.28000E+2, 5.29000E+2, 5.30000E+2, 5.31000E+2, 5.32000E+2, 5.33000E+2, 5.34000E+2, 5.35000E+2, 5.36000E+2, 5.37000E+2, 5.38000E+2, 5.39000E+2, 5.40000E+2, 5.41000E+2, 5.42000E+2, 5.43000E+2, 5.44000E+2, 5.45000E+2, 5.46000E+2, 5.47000E+2, 5.48000E+2, 5.49000E+2, 5.50000E+2, 5.51000E+2, 5.52000E+2, 5.53000E+2, 5.54000E+2, 5.55000E+2, 5.56000E+2, 5.57000E+2, 5.58000E+2, 5.59000E+2, 5.60000E+2, 5.61000E+2, 5.62000E+2, 5.63000E+2, 5.64000E+2, 5.65000E+2, 5.66000E+2, 5.67000E+2, 5.68000E+2, 5.69000E+2, 5.70000E+2, 5.71000E+2, 5.72000E+2, 5.73000E+2, 5.74000E+2, 5.75000E+2, 5.76000E+2, 5.77000E+2, 5.78000E+2, 5.79000E+2, 5.80000E+2, 5.81000E+2, 5.82000E+2, 5.83000E+2, 5.84000E+2, 5.85000E+2, 5.86000E+2, 5.87000E+2, 5.88000E+2, 5.89000E+2, 5.90000E+2, 5.91000E+2, 5.92000E+2, 5.93000E+2, 5.94000E+2, 5.95000E+2, 5.96000E+2, 5.97000E+2, 5.98000E+2, 5.99000E+2, 6.00000E+2, 6.01000E+2, 6.02000E+2, 6.03000E+2, 6.04000E+2, 6.05000E+2, 6.06000E+2, 6.07000E+2, 6.08000E+2, 6.09000E+2, 6.10000E+2, 6.11000E+2, 6.12000E+2, 6.13000E+2, 6.14000E+2, 6.15000E+2, 6.16000E+2, 6.17000E+2, 6.18000E+2, 6.19000E+2, 6.20000E+2, 6.21000E+2, 6.22000E+2, 6.23000E+2, 6.24000E+2, 6.25000E+2, 6.26000E+2, 6.27000E+2, 6.28000E+2, 6.29000E+2, 6.30000E+2, 6.31000E+2, 6.32000E+2, 6.33000E+2, 6.34000E+2, 6.35000E+2, 6.36000E+2, 6.37000E+2, 6.38000E+2, 6.39000E+2, 6.40000E+2, 6.41000E+2, 6.42000E+2, 6.43000E+2, 6.44000E+2, 6.45000E+2, 6.46000E+2, 6.47000E+2, 6.48000E+2, 6.49000E+2, 6.50000E+2, 6.51000E+2, 6.52000E+2, 6.53000E+2, 6.54000E+2, 6.55000E+2, 6.56000E+2, 6.57000E+2, 6.58000E+2, 6.59000E+2, 6.60000E+2, 6.61000E+2, 6.62000E+2, 6.63000E+2, 6.64000E+2, 6.65000E+2, 6.66000E+2, 6.67000E+2, 6.68000E+2, 6.69000E+2, 6.70000E+2, 6.71000E+2, 6.72000E+2, 6.73000E+2, 6.74000E+2, 6.75000E+2, 6.76000E+2, 6.77000E+2, 6.78000E+2, 6.79000E+2, 6.80000E+2, 6.81000E+2, 6.82000E+2, 6.83000E+2, 6.84000E+2, 6.85000E+2, 6.86000E+2, 6.87000E+2, 6.88000E+2, 6.89000E+2, 6.90000E+2, 6.91000E+2, 6.92000E+2, 6.93000E+2, 6.94000E+2, 6.95000E+2, 6.96000E+2, 6.97000E+2, 6.98000E+2, 6.99000E+2, 7.00000E+2, 7.01000E+2, 7.02000E+2, 7.03000E+2, 7.04000E+2, 7.05000E+2, 7.06000E+2, 7.07000E+2, 7.08000E+2, 7.09000E+2, 7.10000E+2, 7.11000E+2, 7.12000E+2, 7.13000E+2, 7.14000E+2, 7.15000E+2, 7.16000E+2, 7.17000E+2, 7.18000E+2, 7.19000E+2, 7.20000E+2, 7.21000E+2, 7.22000E+2, 7.23000E+2, 7.24000E+2, 7.25000E+2, 7.26000E+2, 7.27000E+2, 7.28000E+2, 7.29000E+2, 7.30000E+2, 7.31000E+2, 7.32000E+2, 7.33000E+2, 7.34000E+2, 7.35000E+2, 7.36000E+2, 7.37000E+2, 7.38000E+2, 7.39000E+2, 7.40000E+2, 7.41000E+2, 7.42000E+2, 7.43000E+2, 7.44000E+2, 7.45000E+2, 7.46000E+2, 7.47000E+2, 7.48000E+2, 7.49000E+2, 7.50000E+2, 7.51000E+2, 7.52000E+2, 7.53000E+2, 7.54000E+2, 7.55000E+2, 7.56000E+2, 7.57000E+2, 7.58000E+2, 7.59000E+2, 7.60000E+2, 7.61000E+2, 7.62000E+2, 7.63000E+2, 7.64000E+2, 7.65000E+2, 7.66000E+2, 7.67000E+2, 7.68000E+2, 7.69000E+2, 7.70000E+2, 7.71000E+2, 7.72000E+2, 7.73000E+2, 7.74000E+2, 7.75000E+2, 7.76000E+2, 7.77000E+2, 7.78000E+2, 7.79000E+2, 7.80000E+2, 7.81000E+2, 7.82000E+2, 7.83000E+2, 7.84000E+2, 7.85000E+2, 7.86000E+2, 7.87000E+2, 7.88000E+2, 7.89000E+2, 7.90000E+2, 7.91000E+2, 7.92000E+2, 7.93000E+2, 7.94000E+2, 7.95000E+2, 7.96000E+2, 7.97000E+2, 7.98000E+2, 7.99000E+2, 8.00000E+2, 8.01000E+2, 8.02000E+2, 8.03000E+2, 8.04000E+2, 8.05000E+2, 8.06000E+2, 8.07000E+2, 8.08000E+2, 8.09000E+2, 8.10000E+2, 8.11000E+2, 8.12000E+2, 8.13000E+2, 8.14000E+2, 8.15000E+2, 8.16000E+2, 8.17000E+2, 8.18000E+2, 8.19000E+2, 8.20000E+2, 8.21000E+2, 8.22000E+2, 8.23000E+2, 8.24000E+2, 8.25000E+2, 8.26000E+2, 8.27000E+2, 8.28000E+2, 8.29000E+2, 8.30000E+2, 8.31000E+2, 8.32000E+2, 8.33000E+2, 8.34000E+2, 8.35000E+2, 8.36000E+2, 8.37000E+2, 8.38000E+2, 8.39000E+2, 8.40000E+2, 8.41000E+2, 8.42000E+2, 8.43000E+2, 8.44000E+2, 8.45000E+2, 8.46000E+2, 8.47000E+2, 8.48000E+2, 8.49000E+2, 8.50000E+2, 8.51000E+2, 8.52000E+2, 8.53000E+2, 8.54000E+2, 8.55000E+2, 8.56000E+2, 8.57000E+2, 8.58000E+2, 8.59000E+2, 8.60000E+2, 8.61000E+2, 8.62000E+2, 8.63000E+2, 8.64000E+2, 8.65000E+2, 8.66000E+2, 8.67000E+2, 8.68000E+2, 8.69000E+2, 8.70000E+2, 8.71000E+2, 8.72000E+2, 8.73000E+2, 8.74000E+2, 8.75000E+2, 8.76000E+2, 8.77000E+2, 8.78000E+2, 8.79000E+2, 8.80000E+2, 8.81000E+2, 8.82000E+2, 8.83000E+2, 8.84000E+2, 8.85000E+2, 8.86000E+2, 8.87000E+2, 8.88000E+2, 8.89000E+2, 8.90000E+2, 8.91000E+2, 8.92000E+2, 8.93000E+2, 8.94000E+2, 8.95000E+2, 8.96000E+2, 8.97000E+2, 8.98000E+2, 8.99000E+2, 9.00000E+2, 9.01000E+2, 9.02000E+2, 9.03000E+2, 9.04000E+2, 9.05000E+2, 9.06000E+2, 9.07000E+2, 9.08000E+2, 9.09000E+2, 9.10000E+2, 9.11000E+2, 9.12000E+2, 9.13000E+2, 9.14000E+2, 9.15000E+2, 9.16000E+2, 9.17000E+2, 9.18000E+2, 9.19000E+2, 9.20000E+2, 9.21000E+2, 9.22000E+2, 9.23000E+2, 9.24000E+2, 9.25000E+2, 9.26000E+2, 9.27000E+2, 9.28000E+2, 9.29000E+2, 9.30000E+2, 9.31000E+2, 9.32000E+2, 9.33000E+2, 9.34000E+2, 9.35000E+2, 9.36000E+2, 9.37000E+2, 9.38000E+2, 9.39000E+2, 9.40000E+2, 9.41000E+2, 9.42000E+2, 9.43000E+2, 9.44000E+2, 9.45000E+2, 9.46000E+2, 9.47000E+2, 9.48000E+2, 9.49000E+2, 9.50000E+2, 9.51000E+2, 9.52000E+2, 9.53000E+2, 9.54000E+2, 9.55000E+2, 9.56000E+2, 9.57000E+2, 9.58000E+2, 9.59000E+2, 9.60000E+2, 9.61000E+2, 9.62000E+2, 9.63000E+2, 9.64000E+2, 9.65000E+2, 9.66000E+2, 9.67000E+2, 9.68000E+2, 9.69000E+2, 9.70000E+2, 9.71000E+2, 9.72000E+2, 9.73000E+2, 9.74000E+2, 9.75000E+2, 9.76000E+2, 9.77000E+2, 9.78000E+2, 9.79000E+2, 9.80000E+2, 9.81000E+2, 9.82000E+2, 9.83000E+2, 9.84000E+2, 9.85000E+2, 9.86000E+2, 9.87000E+2, 9.88000E+2, 9.89000E+2, 9.90000E+2, 9.91000E+2, 9.92000E+2, 9.93000E+2, 9.94000E+2, 9.95000E+2, 9.96000E+2, 9.97000E+2, 9.98000E+2, 9.99000E+2, 1.00000E+3, 1.00100E+3, 1.00200E+3, 1.00300E+3, 1.00400E+3, 1.00500E+3, 1.00600E+3, 1.00700E+3, 1.00800E+3, 1.00900E+3, 1.01000E+3, 1.01100E+3, 1.01200E+3, 1.01300E+3, 1.01400E+3, 1.01500E+3, 1.01600E+3, 1.01700E+3, 1.01800E+3, 1.01900E+3, 1.02000E+3, 1.02100E+3, 1.02200E+3, 1.02300E+3, 1.02400E+3, 1.02500E+3, 1.02600E+3, 1.02700E+3, 1.02800E+3, 1.02900E+3, 1.03000E+3, 1.03100E+3, 1.03200E+3, 1.03300E+3, 1.03400E+3, 1.03500E+3, 1.03600E+3, 1.03700E+3, 1.03800E+3, 1.03900E+3, 1.04000E+3, 1.04100E+3, 1.04200E+3, 1.04300E+3, 1.04400E+3, 1.04500E+3, 1.04600E+3, 1.04700E+3, 1.04800E+3, 1.04900E+3, 1.05000E+3, 1.05100E+3, 1.05200E+3, 1.05300E+3, 1.05400E+3, 1.05500E+3, 1.05600E+3, 1.05700E+3, 1.05800E+3, 1.05900E+3, 1.06000E+3, 1.06100E+3, 1.06200E+3, 1.06300E+3, 1.06400E+3, 1.06500E+3, 1.06600E+3, 1.06700E+3, 1.06800E+3, 1.06900E+3, 1.07000E+3, 1.07100E+3, 1.07200E+3, 1.07300E+3, 1.07400E+3, 1.07500E+3, 1.07600E+3, 1.07700E+3, 1.07800E+3, 1.07900E+3, 1.08000E+3, 1.08100E+3, 1.08200E+3, 1.08300E+3, 1.08400E+3, 1.08500E+3, 1.08600E+3, 1.08700E+3, 1.08800E+3, 1.08900E+3, 1.09000E+3, 1.09100E+3, 1.09200E+3, 1.09300E+3, 1.09400E+3, 1.09500E+3, 1.09600E+3, 1.09700E+3, 1.09800E+3, 1.09900E+3, 1.10000E+3, 1.10100E+3, 1.10200E+3, 1.10300E+3, 1.10400E+3, 1.10500E+3, 1.10600E+3, 1.10700E+3, 1.10800E+3, 1.10900E+3, 1.11000E+3, 1.11100E+3, 1.11200E+3, 1.11300E+3, 1.11400E+3, 1.11500E+3, 1.11600E+3, 1.11700E+3, 1.11800E+3, 1.11900E+3, 1.12000E+3, 1.12100E+3, 1.12200E+3, 1.12300E+3, 1.12400E+3, 1.12500E+3, 1.12600E+3, 1.12700E+3, 1.12800E+3, 1.12900E+3, 1.13000E+3, 1.13100E+3, 1.13200E+3, 1.13300E+3, 1.13400E+3, 1.13500E+3, 1.13600E+3, 1.13700E+3, 1.13800E+3, 1.13900E+3, 1.14000E+3, 1.14100E+3, 1.14200E+3, 1.14300E+3, 1.14400E+3, 1.14500E+3, 1.14600E+3, 1.14700E+3, 1.14800E+3, 1.14900E+3, 1.15000E+3, 1.15100E+3, 1.15200E+3, 1.15300E+3, 1.15400E+3, 1.15500E+3, 1.15600E+3, 1.15700E+3, 1.15800E+3, 1.15900E+3, 1.16000E+3, 1.16100E+3, 1.16200E+3, 1.16300E+3, 1.16400E+3, 1.16500E+3, 1.16600E+3, 1.16700E+3, 1.16800E+3, 1.16900E+3, 1.17000E+3, 1.17100E+3, 1.17200E+3, 1.17300E+3, 1.17400E+3, 1.17500E+3, 1.17600E+3, 1.17700E+3, 1.17800E+3, 1.17900E+3, 1.18000E+3, 1.18100E+3, 1.18200E+3, 1.18300E+3, 1.18400E+3, 1.18500E+3, 1.18600E+3, 1.18700E+3, 1.18800E+3, 1.18900E+3, 1.19000E+3, 1.19100E+3, 1.19200E+3, 1.19300E+3, 1.19400E+3, 1.19500E+3, 1.19600E+3, 1.19700E+3, 1.19800E+3, 1.19900E+3, 1.20000E+3, 1.20100E+3, 1.20200E+3, 1.20300E+3, 1.20400E+3, 1.20500E+3, 1.20600E+3, 1.20700E+3, 1.20800E+3, 1.20900E+3, 1.21000E+3, 1.21100E+3, 1.21200E+3, 1.21300E+3, 1.21400E+3, 1.21500E+3, 1.21600E+3, 1.21700E+3, 1.21800E+3, 1.21900E+3, 1.22000E+3, 1.22100E+3, 1.22200E+3, 1.22300E+3, 1.22400E+3, 1.22500E+3, 1.22600E+3, 1.22700E+3, 1.22800E+3, 1.22900E+3, 1.23000E+3, 1.23100E+3, 1.23200E+3, 1.23300E+3, 1.23400E+3, 1.23500E+3, 1.23600E+3, 1.23700E+3, 1.23800E+3, 1.23900E+3, 1.24000E+3, 1.24100E+3, 1.24200E+3, 1.24300E+3, 1.24400E+3, 1.24500E+3, 1.24600E+3, 1.24700E+3, 1.24800E+3, 1.24900E+3, 1.25000E+3, 1.25100E+3, 1.25200E+3, 1.25300E+3, 1.25400E+3, 1.25500E+3, 1.25600E+3, 1.25700E+3, 1.25800E+3, 1.25900E+3, 1.26000E+3, 1.26100E+3, 1.26200E+3, 1.26300E+3, 1.26400E+3, 1.26500E+3, 1.26600E+3, 1.26700E+3, 1.26800E+3, 1.26900E+3, 1.27000E+3, 1.27100E+3, 1.27200E+3, 1.27300E+3, 1.27400E+3, 1.27500E+3, 1.27600E+3, 1.27700E+3, 1.27800E+3, 1.27900E+3, 1.28000E+3, 1.28100E+3, 1.28200E+3, 1.28300E+3, 1.28400E+3, 1.28500E+3, 1.28600E+3, 1.28700E+3, 1.28800E+3, 1.28900E+3, 1.29000E+3, 1.29100E+3, 1.29200E+3, 1.29300E+3, 1.29400E+3, 1.29500E+3, 1.29600E+3, 1.29700E+3, 1.29800E+3, 1.29900E+3, 1.30000E+3, 1.30100E+3, 1.30200E+3, 1.30300E+3, 1.30400E+3, 1.30500E+3, 1.30600E+3, 1.30700E+3, 1.30800E+3, 1.30900E+3, 1.31000E+3, 1.31100E+3, 1.31200E+3, 1.31300E+3, 1.31400E+3, 1.31500E+3, 1.31600E+3, 1.31700E+3, 1.31800E+3, 1.31900E+3, 1.32000E+3, 1.32100E+3, 1.32200E+3, 1.32300E+3, 1.32400E+3, 1.32500E+3, 1.32600E+3, 1.32700E+3, 1.32800E+3, 1.32900E+3, 1.33000E+3, 1.33100E+3, 1.33200E+3, 1.33300E+3, 1.33400E+3, 1.33500E+3, 1.33600E+3, 1.33700E+3, 1.33800E+3, 1.33900E+3, 1.34000E+3, 1.34100E+3, 1.34200E+3, 1.34300E+3, 1.34400E+3, 1.34500E+3, 1.34600E+3, 1.34700E+3, 1.34800E+3, 1.34900E+3, 1.35000E+3, 1.35100E+3, 1.35200E+3, 1.35300E+3, 1.35400E+3, 1.35500E+3, 1.35600E+3, 1.35700E+3, 1.35800E+3, 1.35900E+3, 1.36000E+3, 1.36100E+3, 1.36200E+3, 1.36300E+3, 1.36400E+3, 1.36500E+3, 1.36600E+3, 1.36700E+3, 1.36800E+3, 1.36900E+3, 1.37000E+3, 1.37100E+3, 1.37200E+3, 1.37300E+3, 1.37400E+3, 1.37500E+3, 1.37600E+3, 1.37700E+3, 1.37800E+3, 1.37900E+3, 1.38000E+3, 1.38100E+3, 1.38200E+3, 1.38300E+3, 1.38400E+3, 1.38500E+3, 1.38600E+3, 1.38700E+3, 1.38800E+3, 1.38900E+3, 1.39000E+3, 1.39100E+3, 1.39200E+3, 1.39300E+3, 1.39400E+3, 1.39500E+3, 1.39600E+3, 1.39700E+3, 1.39800E+3, 1.39900E+3, 1.40000E+3, 1.40100E+3, 1.40200E+3, 1.40300E+3, 1.40400E+3, 1.40500E+3, 1.40600E+3, 1.40700E+3, 1.40800E+3, 1.40900E+3, 1.41000E+3, 1.41100E+3, 1.41200E+3, 1.41300E+3, 1.41400E+3, 1.41500E+3, 1.41600E+3, 1.41700E+3, 1.41800E+3, 1.41900E+3, 1.42000E+3, 1.42100E+3, 1.42200E+3, 1.42300E+3, 1.42400E+3, 1.42500E+3, 1.42600E+3, 1.42700E+3, 1.42800E+3, 1.42900E+3, 1.43000E+3, 1.43100E+3, 1.43200E+3, 1.43300E+3, 1.43400E+3, 1.43500E+3, 1.43600E+3, 1.43700E+3, 1.43800E+3, 1.43900E+3, 1.44000E+3, 1.44100E+3, 1.44200E+3, 1.44300E+3, 1.44400E+3, 1.44500E+3, 1.44600E+3, 1.44700E+3, 1.44800E+3, 1.44900E+3, 1.45000E+3, 1.45100E+3, 1.45200E+3, 1.45300E+3, 1.45400E+3, 1.45500E+3, 1.45600E+3, 1.45700E+3, 1.45800E+3, 1.45900E+3, 1.46000E+3, 1.46100E+3, 1.46200E+3, 1.46300E+3, 1.46400E+3, 1.46500E+3, 1.46600E+3, 1.46700E+3, 1.46800E+3, 1.46900E+3, 1.47000E+3, 1.47100E+3, 1.47200E+3, 1.47300E+3, 1.47400E+3, 1.47500E+3, 1.47600E+3, 1.47700E+3, 1.47800E+3, 1.47900E+3, 1.48000E+3, 1.48100E+3, 1.48200E+3, 1.48300E+3, 1.48400E+3, 1.48500E+3, 1.48600E+3, 1.48700E+3, 1.48800E+3, 1.48900E+3, 1.49000E+3, 1.49100E+3, 1.49200E+3, 1.49300E+3, 1.49400E+3, 1.49500E+3, 1.49600E+3, 1.49700E+3, 1.49800E+3, 1.49900E+3);"
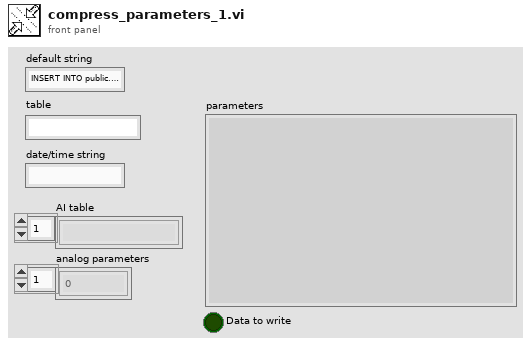
[diagram p1: front panel]
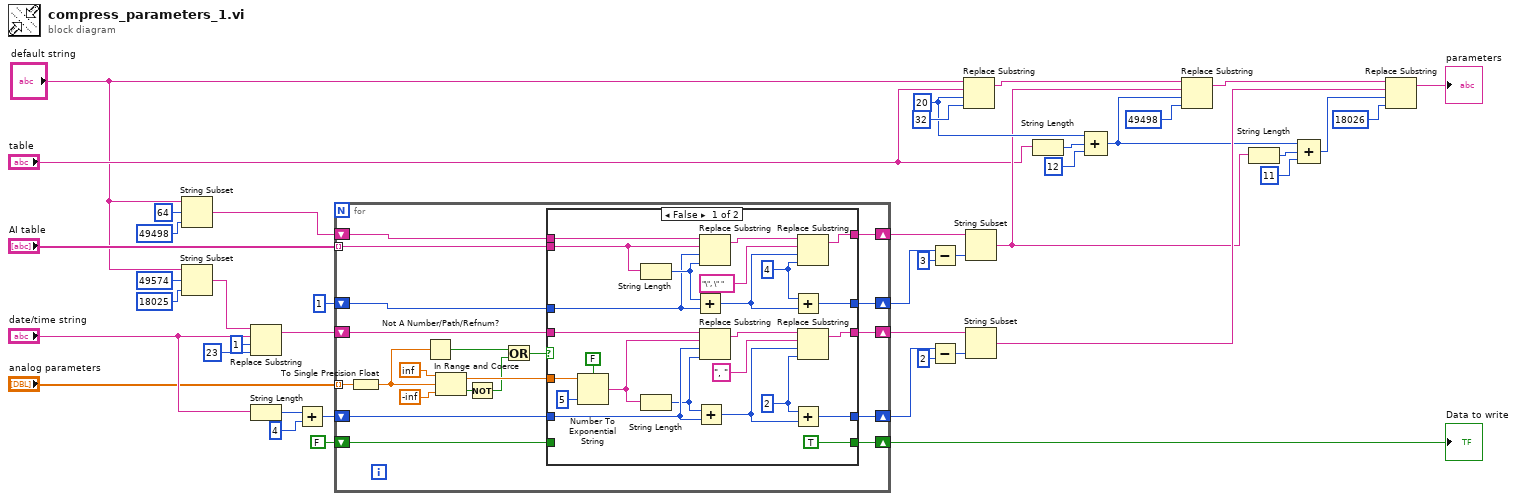
[diagram p0: block diagram]
diagram:
  w35 = 20 ("offset (0)")
  n1 = String Subset(string="default string", offset (0)=64, length (rest)=49498 ("length (rest)")) -> (substring=w19:string)
  n2 = String Subset(string="default string", offset (0)=49574, length (rest)=18025 ("length (rest)")) -> (substring=w7:string)
  n3 = Replace Substring(2:23 ("length (len. of substring)"), 3:1 ("offset (0)"), 4:"date/time string", 5:w7) -> (1:w6:string)  [unwired: 1 out]
  n4 = String Length(string="date/time string") -> (length=w4:i32)
  n5 = Add(x=w4, y=4) -> (x+y=w2:i32)
  n6 = for {
    tunnel: "analog parameters" -> [w45] mode=indexing
    shift-right: [w56] -> w40
    shift-left: w6 -> [w58]
    shift-right: [w57] -> w12
    shift-left: w2 -> [w55]
    tunnel: "AI table" -> [w62] mode=indexing
    shift-right: [w61] -> w17
    shift-left: 1 -> [w59]
    shift-right: [w60] -> w23
    shift-left: w19 -> [w63]
    shift-right: [w47] -> w11
    shift-left: FALSE -> [w46]
    n7 = To Single Precision Float(number=w45) -> (single precision float=w44:sgl)
    n8 = Not A Number/Path/Refnum?(number/path/refnum=w44) -> (NaN/Path/Refnum?=w54:bool)
    n9 = In Range and Coerce(upper limit=sgl inf, x=w44, lower limit=sgl -inf) -> (coerced(x)=w53:sgl, In Range?=w50:bool)
    n10 = Not(x=w50) -> (.not. x?=w49:bool)
    n11 = Or(x=w54, y=w49) -> (x .or. y?=w48:bool)
    n12 = case shown="False" w48 {
      tunnel: w63 -> [w87 w92]
      tunnel: w62 -> [w86 _]
      tunnel: [w80 w91] -> w61
      tunnel: [w79 w92] -> w60
      tunnel: w59 -> [w78 w91]
      tunnel: w58 -> [w74 w90]
      tunnel: [w72 w89] -> w57
      tunnel: [w71 w90] -> w56
      tunnel: w55 -> [w70 w89]
      tunnel: w53 -> [w67 _]
      tunnel: [TRUE w88] -> w47
      tunnel: w46 -> [_ w88]
      frame False {
        w77 = 2 ("x+y")
        w81 = 4 ("x+y")
        n13 = Number To Exponential String(number=w67, precision (6)=i16 5, 1:FALSE ("use system decimal point (T)")) -> (E-format string=w69:string)  [unwired: 1 in]
        n14 = String Length(string=w86) -> (length=w85:i32)
        n15 = String Length(string=w69) -> (length=w68:i32)
        n16 = Add(x=w85, y=w78) -> (x+y=w82:i32)
        n17 = Add(x=w68, y=w70) -> (x+y=w73:i32)
        n18 = Replace Substring(2:w85, 3:w78, 4:w86, 5:w87) -> (1:w84:string)  [unwired: 1 out]
        n19 = Replace Substring(2:w68, 3:w70, 4:w69, 5:w74) -> (1:w75:string)  [unwired: 1 out]
        n20 = Add(x=w81, y=w82) -> (x+y=w80:i32)
        n21 = Add(x=w77, y=w73) -> (x+y=w72:i32)
        n22 = Replace Substring(2:w81, 3:w82, 4:"\", \" ", 5:w84) -> (1:w79:string)  [unwired: 1 out]
        n23 = Replace Substring(2:w77, 3:w73, 4:", ", 5:w75) -> (1:w71:string)  [unwired: 1 out]
      }
      frame True {
      }
    }
  }
  "Data to write" <- w11
  n24 = Subtract(x=w17, y=3) -> (x-y=w16:i32)
  n25 = Subtract(x=w12, y=2) -> (x-y=w42:i32)
  n26 = Replace Substring(2:32 ("length (len. of substring)"), 3:w35, 4:"table", 5:"default string") -> (1:w37:string)  [unwired: 1 out]
  n27 = String Subset(string=w23, length (rest)=w16) -> (substring=w27:string)  [unwired: 1 in]
  n28 = String Subset(string=w40, length (rest)=w42) -> (substring=w32:string)  [unwired: 1 in]
  n29 = String Length(string="table") -> (length=w34:i32)
  n30 = Compound Arithmetic op=ADD(w35, w34, 12 ("value")) -> (w31:i32)
  n31 = Replace Substring(2:49498 ("length (len. of substring)"), 3:w31, 4:w27, 5:w37) -> (1:w33:string)  [unwired: 1 out]
  n32 = String Length(string=w27) -> (length=w30:i32)
  n33 = Compound Arithmetic op=ADD(w31, w30, 11 ("value")) -> (w28:i32)
  n34 = Replace Substring(2:18026 ("length (len. of substring)"), 3:w28, 4:w32, 5:w33) -> (1:→"parameters":string)  [unwired: 1 out]
